vi "RT_MAIN.vi"() -> ()   [LabVIEW 2019]
uses:
  <vilib>/rvi/interface/nirviOpenFPGA/nirviOpenFPGA.xnode
  <vilib>/rvi/interface/nirviMethod/nirviMethod.xnode
  <vilib>/FPGAPlugInAG/Dynamic/niLvFpga_Reset_Dynamic.vi
  <vilib>/FPGAPlugInAG/Dynamic/niLvFpga_Run_Dynamic.vi
  <vilib>/Platform/TimedLoop/XDataNode/XDataNode.xnode
  <vilib>/Platform/TimedLoop/XDataNode/nitl_modes.ctl
  <vilib>/Platform/TimedLoop/XDataNode/XDNodeRunTimeDep.lvlib
  <vilib>/Platform/TimedLoop/XDataNode/wakeup.ctl
  <vilib>/Platform/TimedLoop/XDataNode/timing_clust.ctl
  <vilib>/NI_Real-Time Target Support.lvlib
  <vilib>/FPGAPlugInAG/Dynamic/niLvFpga_Abort_Dynamic.vi
  <vilib>/rvi/interface/nirviCloseFPGA/nirviCloseFPGA.xnode
  ELMO/Elmo Status.ctl
  <vilib>/rvi/interface/nirviReadWriteControl/nirviReadWriteControl.xnode
  <vilib>/Utility/error.llb/Error Cluster From Error Code.vi
  <vilib>/rvi/interface/Simulation/niFpgaSimulationCallBeginRW.vi
  <vilib>/rvi/errors/niLvFpgaAdjustHostInterfaceError.vi
  NiFpgaLv.dll
  <vilib>/Analysis/NI_AALPro.lvlib
  <vilib>/Analysis/5stat.llb/RMS (DBL).vi
  <vilib>/FPGAPlugInAG/Dynamic/niLvFpga_Close_Dynamic.vi
  FPGA Bitfiles/hipabfccurrentpd_FPGATarget_FPGADATA_BIuapcLYHzU.lvbitx
  FPGA/FPGA_DATA.vi
  <vilib>/FPGAPlugInAG/cRIO-9040/niLvFpga_Open_cRIO-9040.vi
  <vilib>/rvi/interface/common/dynamic/niFpgaDynamicAddResources.vi
panel:
  in  "threshold":T1={"High 검출값"=400.0, "Low 기준값"=-400.0, "MID 중간값"=-200.0}
  out "Q_gcp":i32
  out "Control state":string
  in  "문자열":string="system_211111_"
  out "Initial_IMU_R":sgl
  out "Initial_IMU_L":sgl
  out "GCP_R":sgl(slide) scale=0.0..100.0
  out "R_NUM":u32
  in  "Sync Q":bool
  in  "Profile":enum16{"p0", "p1", "p2", "p3", "p4"}(ring)
  in  "Force_peak_control":sgl=300.0
  out "웨이브폼 차트 4":T2(graph)
  out "웨이브폼 차트 3":dbl(graph)
  out "큐의 원소 개수 2":i32
  out "큐의 원소 개수":i32
  out "Q_PSD":i32
  in  "Tuning  2":bool
  out "웨이브폼 차트 2":T3(graph)
  in  "Base force":sgl
  in  "Force_peak":sgl
  in  "ILC coefficient":sgl=0.01
  out "웨이브폼 차트":T3(graph)
  out "Q_motor":i32
  out "Q_data":i32
  out "Q_motor":i32
  out "Status_PS":string
  out "Control param In":T4
  in  "Current Limid 1":cluster{"output high":dbl, "output low":dbl}={"output high"=2885.0, "output low"=-2885.0} {"output high" format="%.2f"; "output low" format="%.2f"}
  in  "Force PD":T5={"proportional gain (Kc)"=15.0, "integral time (Ti, min)"=0.0, "derivative time (Td, min)"=0.0001700000000000005} caption="Force PD 1" {"proportional gain (Kc)" format="%.7f"; "integral time (Ti, min)" format="%.7f"; "derivative time (Td, min)" format="%.7f"}
  in  "2 On/ 1 Off 2":bool
  in  "Motor 0 on / 1 off 2":bool
  in  "PID Set Time(ms) 2":i32
  in  "Force PD":cluster{"(Kp)":dbl, "(Ti)":dbl, "(Td)":dbl}={"(Kp)"=15.0, "(Ti)"=0.0, "(Td)"=0.0002} caption="Force PD 0" {"(Kp)" format="%.7f"; "(Ti)" format="%.7f"; "(Td)" format="%.7f"}
  in  "Current Limd 0":cluster{"output high":dbl, "output low":dbl}={"output high"=2885.0, "output low"=-2885.0} {"output high" format="%.2f"; "output low" format="%.2f"}
  out "A_vel_1":i32
  out "A_pos_1":i32
  out "A Vel_0":i32
  out "A_Pos_0":i32
  out "Motor state":T6(ring)
  in  "SAVE":bool
  out "CPU_LOAD_0 (%)":dbl format="%#_3g"
  out "CPU_LOAD_1 (%)":dbl format="%#_3g"
  in  "STOP":bool
  # "0이 오른쪽 \n1이 왼쪽"
  # "15\n0.0002"
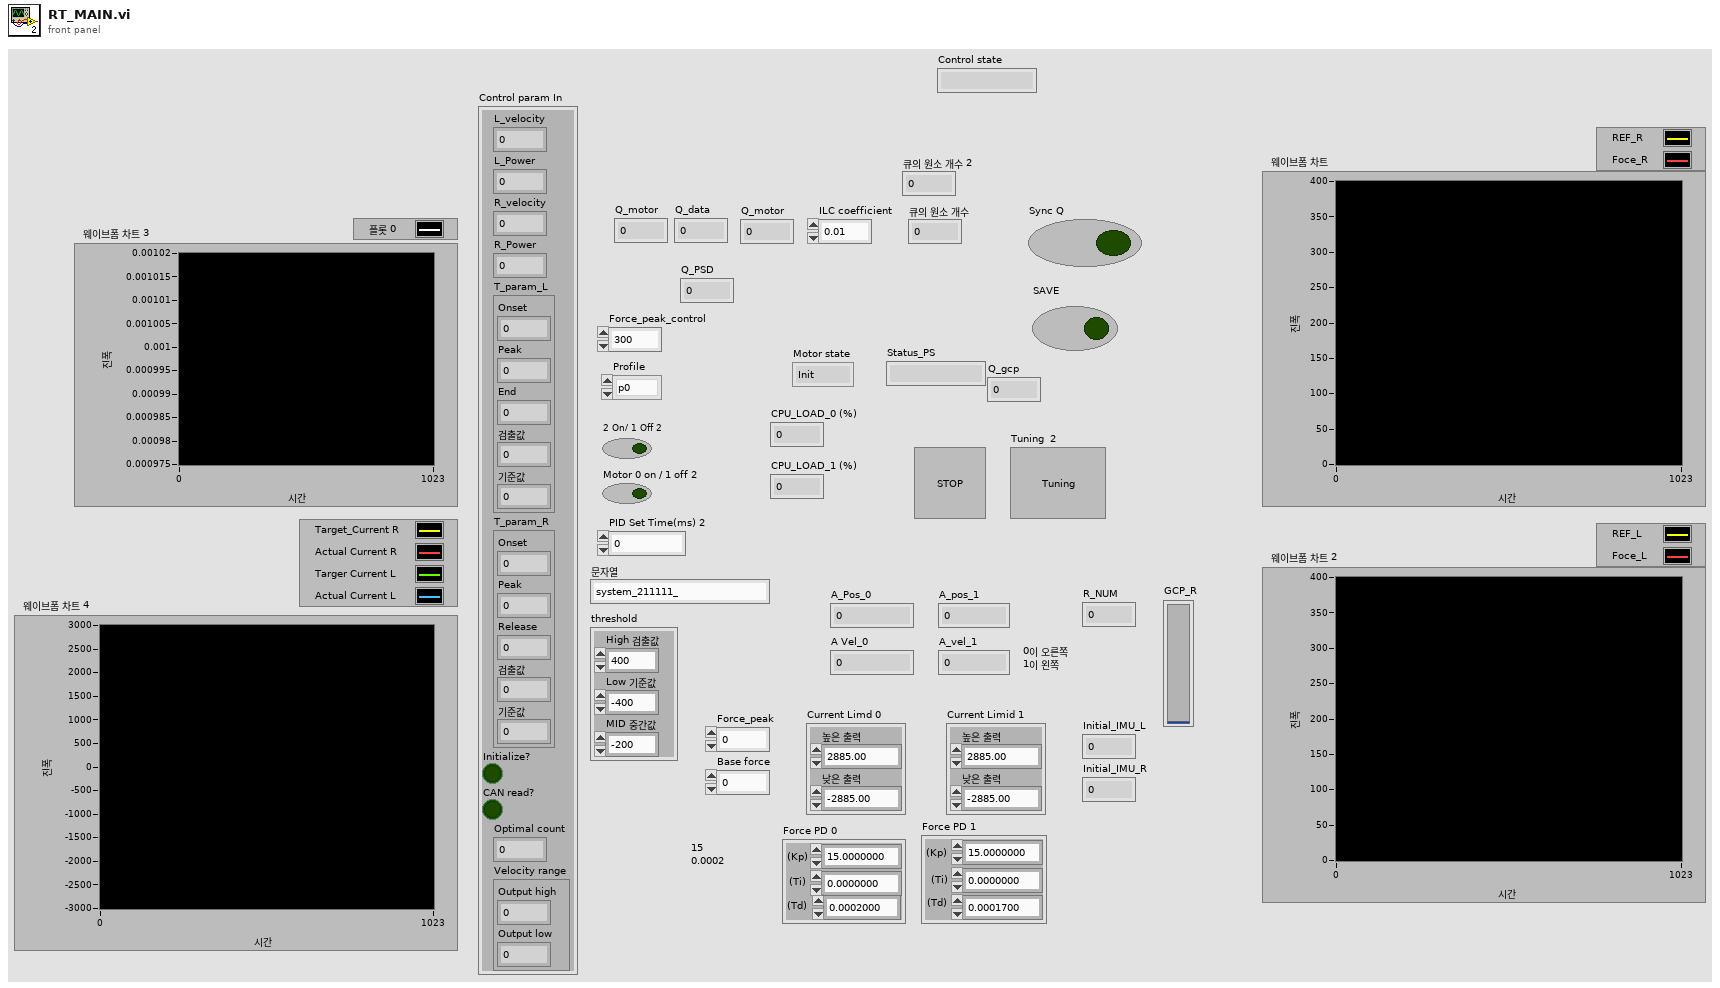
[diagram p1: front panel]
types:
  T1 = cluster{"High 검출값":sgl, "Low 기준값":sgl, "MID 중간값":sgl}
  T2 = cluster{"current_R":i32, "Target Pos_0":i32, "current_L":i32, "Target Pos_0":i32}
  T3 = cluster{"Reference force R":dbl, "Reference force R":dbl}
  T4 = cluster{"L_velocity":u32, "L_Power":sgl, "R_velocity":u32, "R_Power":sgl, "T_param_L":cluster{"Onset":sgl, "Peak":sgl, "End":sgl, "검출값":sgl, "기준값":sgl}, "T_param_R":cluster{"Onset":sgl, "Peak":sgl, "Release":sgl, "검출값":sgl, "기준값":sgl}, "Initialize?":bool, "CAN read?":bool, "Optimal count":i32, "Velocity range":cluster{"Output high":dbl, "Output low":dbl}}
  T5 = cluster{"proportional gain (Kc)":dbl, "integral time (Ti, min)":dbl, "derivative time (Td, min)":dbl}
  T6 = enum16{"Init", "ChkRdy", "Snyc", "Tuning", "Manual"}
  T7 = typedef "XDNodeRunTimeDep.lvlib/timing_clust.ctl" = cluster{"Expected End [f-1]":u64, "Actual End [f-1]":u64, "Finished Late? [f-1]":bool, "Expected End [i-1]":u64, "Actual End [i-1]":u64, "Finished Late? [i-1]":bool, "Expected Start [i]":u64, "Actual Start [i]":u64, "Expected Start [f]":u64, "Actual Start [f]":u64, "Source Name":string, "Structure Name":string, "Period":i64, "Deadline":i64, "Offset":i64, "Start":i64, "Priority":i32, "Timeout":i32, "Mode":T8, "Wakeup Reason":T9, "Error":errorcluster, "Source Type":string, "Secondary Source Type":string, "Global End Time":u64, "Global Start Time":u64, "Frame Duration":u64, "Iteration Duration":u64, "Assigned CPU":i32, "I/O Scan Engine Mode":u32}
  T8 = typedef "XDNodeRunTimeDep.lvlib/nitl_modes.ctl" = enum32{"No Change", "Process missed periods, maintain original phase", "Discard missed periods, maintain original phase", "Process missed periods, ignore original phase", "Discard missed periods, ignore original phase"}
  T9 = typedef "XDNodeRunTimeDep.lvlib/wakeup.ctl" = enum32{"Normal", "Aborted", "Asynchronous wakeup", "Timing source error", "Timed loop error", "Timeout"}
  T10 = typedef "Elmo Status.ctl" = enum16{"Not ready to switch on", "Switch on disabled", "Ready to switch on", "Switch on", "Operation Enabled", "Quick stop active", "Fault reaction active", "Fault", "None"}
  T11 = enum16{"open", "replace", "create", "open or create", "replace or create", "replace or create with confirmation"}
  T12 = cluster{"R_angvel_raw":sgl, "R_angvel_filt":sgl, "L_angvel_raw":sgl, "L_angvel_filt":sgl, "Q_GCP":cluster{"L_num":u32, "L_GCP":dbl, "L_Period":u32, "R_num":u32, "R_GCP":dbl, "R_Period":u32, "L_Ctrl_St":bool, "R_Ctrl_St":bool}}
  T13 = cluster{"L_num":u32, "L_GCP":dbl, "L_Period":u32, "R_num":u32, "R_GCP":dbl, "R_Period":u32, "L_Ctrl_St":bool, "R_Ctrl_St":bool}
  T14 = cluster{"LOAD_CELL_PEAK_L":sgl[], "LOAD_CELL_PEAK_R":sgl[], "Flag_L":enum16{"Release_start", "Calculate", "Onset_start", "Peak_start"}, "Flag_R":enum16{"Release_start", "Calculate", "Onset_start", "Peak_start"}, "Status_PS":string, "GCP_1k_R":sgl, "GCP_1k_L":sgl}
  T15 = cluster{"Actual Pos_0":i32, "Actual Vel_0":i32, "Target Cur_0":i32, "Actual Cur_0":i32, "Actual Pos_1":i32, "Actual Vel_1":i32, "Target Cur_1":i32, "Actual Cur_1":i32, "status_0 ":u16, "status_1":u16}
  T16 = cluster{"Num_L":u32, "Period_L":u32, "GCP_L":sgl, "Num_R":u32, "Period_R":u32, "GCP_R":sgl, "FPGA_Data":sgl[], "L_RUN_OK":bool, "R_RUN_OK":bool, "L_ctrl_start":bool, "R_ctrl_start":bool, "Loop time":dbl, "Integrated time":dbl, "Mode":enum16{"Negative", "Positive", "Full"}}
  T17 = cluster{"Status_PS":string, "Q to xsensor":bool, "FPGA_data":sgl[], "R_force":sgl, "L_force":sgl, "Param":cluster{"Init_Onset_Load":sgl, "Pos_base_L":sgl, "Pos_base_R":sgl, "Init_Vel":i32, "Init_Accel":u32, "Test_Vel":i32, "Test_Acc":u32, "Load_Warning":sgl, "Load_Alarm":sgl, "Control param In":cluster{"L_velocity":u32, "L_Power":sgl, "R_velocity":u32, "R_Power":sgl, "T_param_L":cluster{"Onset":sgl, "Peak":sgl, "End":sgl, "검출값":sgl, "기준값":sgl}, "T_param_R":cluster{"Onset":sgl, "Peak":sgl, "Release":sgl, "검출값":sgl, "기준값":sgl}, "Initialize?":bool, "CAN read?":bool, "Optimal count":i32, "Velocity range":cluster{"Output high":dbl, "Output low":dbl}}, "Init_R":bool, "Init_L":bool, "Force_mode_R":bool, "Force mode_L":bool, "GCP_L":sgl, "GCP_R":sgl, "D_Vel_L":sgl, "D_Vel_R":sgl, "D_Cur_L(/1000)":sgl, "D_Cur_R(/1000)":sgl, "Force_reference_L":sgl, "Force_reference_R":sgl, "Initial_IMU_L":sgl, "Initial_IMU_R":sgl, "L_NUM":u32, "L_Period":i16, "R_NUM":u32, "R_Period":i16, "Initialization count":i32, "R_Ctrl_St":bool, "L_Ctrl_St":bool}}
  T18 = cluster{"Cmd":string, "PSD_state":string, "R_NUM":u32, "L_NUM":u32, "Force_ref_R":sgl, "Force_ref_L":sgl, "Force_L":sgl, "Force_R":sgl, "Force_Mode_R ":bool, "Force_Mode_L":bool, "Current range":cluster{"output high":dbl, "output low":dbl}}
  T19 = cluster{"output high":dbl, "output low":dbl, "proportional gain (Kc)":dbl, "integral time (Ti, min)":dbl, "derivative time (Td, min)":dbl, "output high":dbl, "output low":dbl, "proportional gain (Kc)":dbl, "integral time (Ti, min)":dbl, "derivative time (Td, min)":dbl}
  T20 = cluster{"Q_motor":cluster{"Actual Pos_0":i32, "Actual Vel_0":i32, "Target Cur_0":i32, "Actual Cur_0":i32, "Actual Pos_1":i32, "Actual Vel_1":i32, "Target Cur_1":i32, "Actual Cur_1":i32, "status_0 ":u16, "status_1":u16}, "Q_PSDtoSAVE":i32, "Q_MOTORtoSAVE":i32, "Save_Loop time":dbl, "Save_Integrated time":dbl, "Process":cluster{"Status_PS":string, "Q to xsensor":bool, "FPGA_data":sgl[], "R_force":sgl, "L_force":sgl, "Param":cluster{"Init_Onset_Load":sgl, "Pos_base_L":sgl, "Pos_base_R":sgl, "Init_Vel":i32, "Init_Accel":u32, "Test_Vel":i32, "Test_Acc":u32, "Load_Warning":sgl, "Load_Alarm":sgl, "Control param In":cluster{"L_velocity":u32, "L_Power":sgl, "R_velocity":u32, "R_Power":sgl, "T_param_L":cluster{"Onset":sgl, "Peak":sgl, "End":sgl, "검출값":sgl, "기준값":sgl}, "T_param_R":cluster{"Onset":sgl, "Peak":sgl, "Release":sgl, "검출값":sgl, "기준값":sgl}, "Initialize?":bool, "CAN read?":bool, "Optimal count":i32, "Velocity range":cluster{"Output high":dbl, "Output low":dbl}}, "Init_R":bool, "Init_L":bool, "Force_mode_R":bool, "Force mode_L":bool, "GCP_L":sgl, "GCP_R":sgl, "D_Vel_L":sgl, "D_Vel_R":sgl, "D_Cur_L(/1000)":sgl, "D_Cur_R(/1000)":sgl, "Force_reference_L":sgl, "Force_reference_R":sgl, "Initial_IMU_L":sgl, "Initial_IMU_R":sgl, "L_NUM":u32, "L_Period":i16, "R_NUM":u32, "R_Period":i16, "Initialization count":i32, "R_Ctrl_St":bool, "L_Ctrl_St":bool}}, "GCP":cluster{"R_angvel_raw":sgl, "R_angvel_filt":sgl, "L_angvel_raw":sgl, "L_angvel_filt":sgl, "Q_GCP":cluster{"L_num":u32, "L_GCP":dbl, "L_Period":u32, "R_num":u32, "R_GCP":dbl, "R_Period":u32, "L_Ctrl_St":bool, "R_Ctrl_St":bool}}, "Q_GCPtoSAVE":i32, "Save_loop":i64}
  T21 = cluster{"Q_motor":cluster{"Actual Pos_0":i32, "Actual Vel_0":i32, "Target Cur_0":i32, "Actual Cur_0":i32, "Actual Pos_1":i32, "Actual Vel_1":i32, "Target Cur_1":i32, "Actual Cur_1":i32, "status_0 ":u16, "status_1":u16}, "Q_PSDtoSAVE":i32, "Q_MOTORtoSAVE":i32, "Save_Loop time":dbl, "Save_Integrated time":dbl, "Process":cluster{"Status_PS":string, "Q to xsensor":bool, "FPGA_data":sgl[], "R_force":sgl, "L_force":sgl, "Param":cluster{"Init_Onset_Load":sgl, "Pos_base_L":sgl, "Pos_base_R":sgl, "Init_Vel":i32, "Init_Accel":u32, "Test_Vel":i32, "Test_Acc":u32, "Load_Warning":sgl, "Load_Alarm":sgl, "Control param In":cluster{"L_velocity":u32, "L_Power":sgl, "R_velocity":u32, "R_Power":sgl, "T_param_L":cluster{"Onset":sgl, "Peak":sgl, "End":sgl, "검출값":sgl, "기준값":sgl}, "T_param_R":cluster{"Onset":sgl, "Peak":sgl, "Release":sgl, "검출값":sgl, "기준값":sgl}, "Initialize?":bool, "CAN read?":bool, "Optimal count":i32, "Velocity range":cluster{"Output high":dbl, "Output low":dbl}}, "Init_R":bool, "Init_L":bool, "Force_mode_R":bool, "Force mode_L":bool, "GCP_L":sgl, "GCP_R":sgl, "D_Vel_L":sgl, "D_Vel_R":sgl, "D_Cur_L(/1000)":sgl, "D_Cur_R(/1000)":sgl, "Force_reference_L":sgl, "Force_reference_R":sgl, "Initial_IMU_L":sgl, "Initial_IMU_R":sgl, "L_NUM":u32, "L_Period":i16, "R_NUM":u32, "R_Period":i16, "Initialization count":i32, "R_Ctrl_St":bool, "L_Ctrl_St":bool}}, "GCP":cluster{"R_angvel_raw":sgl, "R_angvel_filt":sgl, "L_angvel_raw":sgl, "L_angvel_filt":sgl, "Q_GCP":cluster{"L_num":u32, "L_GCP":dbl, "L_Period":u32, "R_num":u32, "R_GCP":dbl, "R_Period":u32, "L_Ctrl_St":bool, "R_Ctrl_St":bool}}, "Q_GCPtoSAVE":i32, "Save_loop":i64}[]
  T22 = cluster{"Init_Onset_Load":sgl, "Pos_base_L":sgl, "Pos_base_R":sgl, "Init_Vel":i32, "Init_Accel":u32, "Test_Vel":i32, "Test_Acc":u32, "Load_Warning":sgl, "Load_Alarm":sgl, "Control param In":cluster{"L_velocity":u32, "L_Power":sgl, "R_velocity":u32, "R_Power":sgl, "T_param_L":cluster{"Onset":sgl, "Peak":sgl, "End":sgl, "검출값":sgl, "기준값":sgl}, "T_param_R":cluster{"Onset":sgl, "Peak":sgl, "Release":sgl, "검출값":sgl, "기준값":sgl}, "Initialize?":bool, "CAN read?":bool, "Optimal count":i32, "Velocity range":cluster{"Output high":dbl, "Output low":dbl}}, "Init_R":bool, "Init_L":bool, "Force_mode_R":bool, "Force mode_L":bool, "GCP_L":sgl, "GCP_R":sgl, "D_Vel_L":sgl, "D_Vel_R":sgl, "D_Cur_L(/1000)":sgl, "D_Cur_R(/1000)":sgl, "Force_reference_L":sgl, "Force_reference_R":sgl, "Initial_IMU_L":sgl, "Initial_IMU_R":sgl, "L_NUM":u32, "L_Period":i16, "R_NUM":u32, "R_Period":i16, "Initialization count":i32, "R_Ctrl_St":bool, "L_Ctrl_St":bool}
  T23 = typedef "NI_Real-Time Target Support.lvlib/RT CPU Load.ctl" = cluster{"Total (%)":dbl, "Time Critical (%)":dbl, "Timed Structures (%)":dbl, "High (%)":dbl, "Above Normal (%)":dbl, "Normal (%)":dbl, "Background (%)":dbl, "Idle (%)":dbl, "ISR (%)":dbl}
  T24 = cluster{"CPU loads[0]":T23, "CPU loads[1]":T23, "CPU loads[2]":T23, "CPU loads[3]":T23, "CPU loads[4]":T23, "CPU loads[5]":T23, "CPU loads[6]":T23, "CPU loads[7]":T23, "CPU loads[8]":T23}
  T25 = cluster{"Reference force_L":dbl, "Reference force R":dbl}
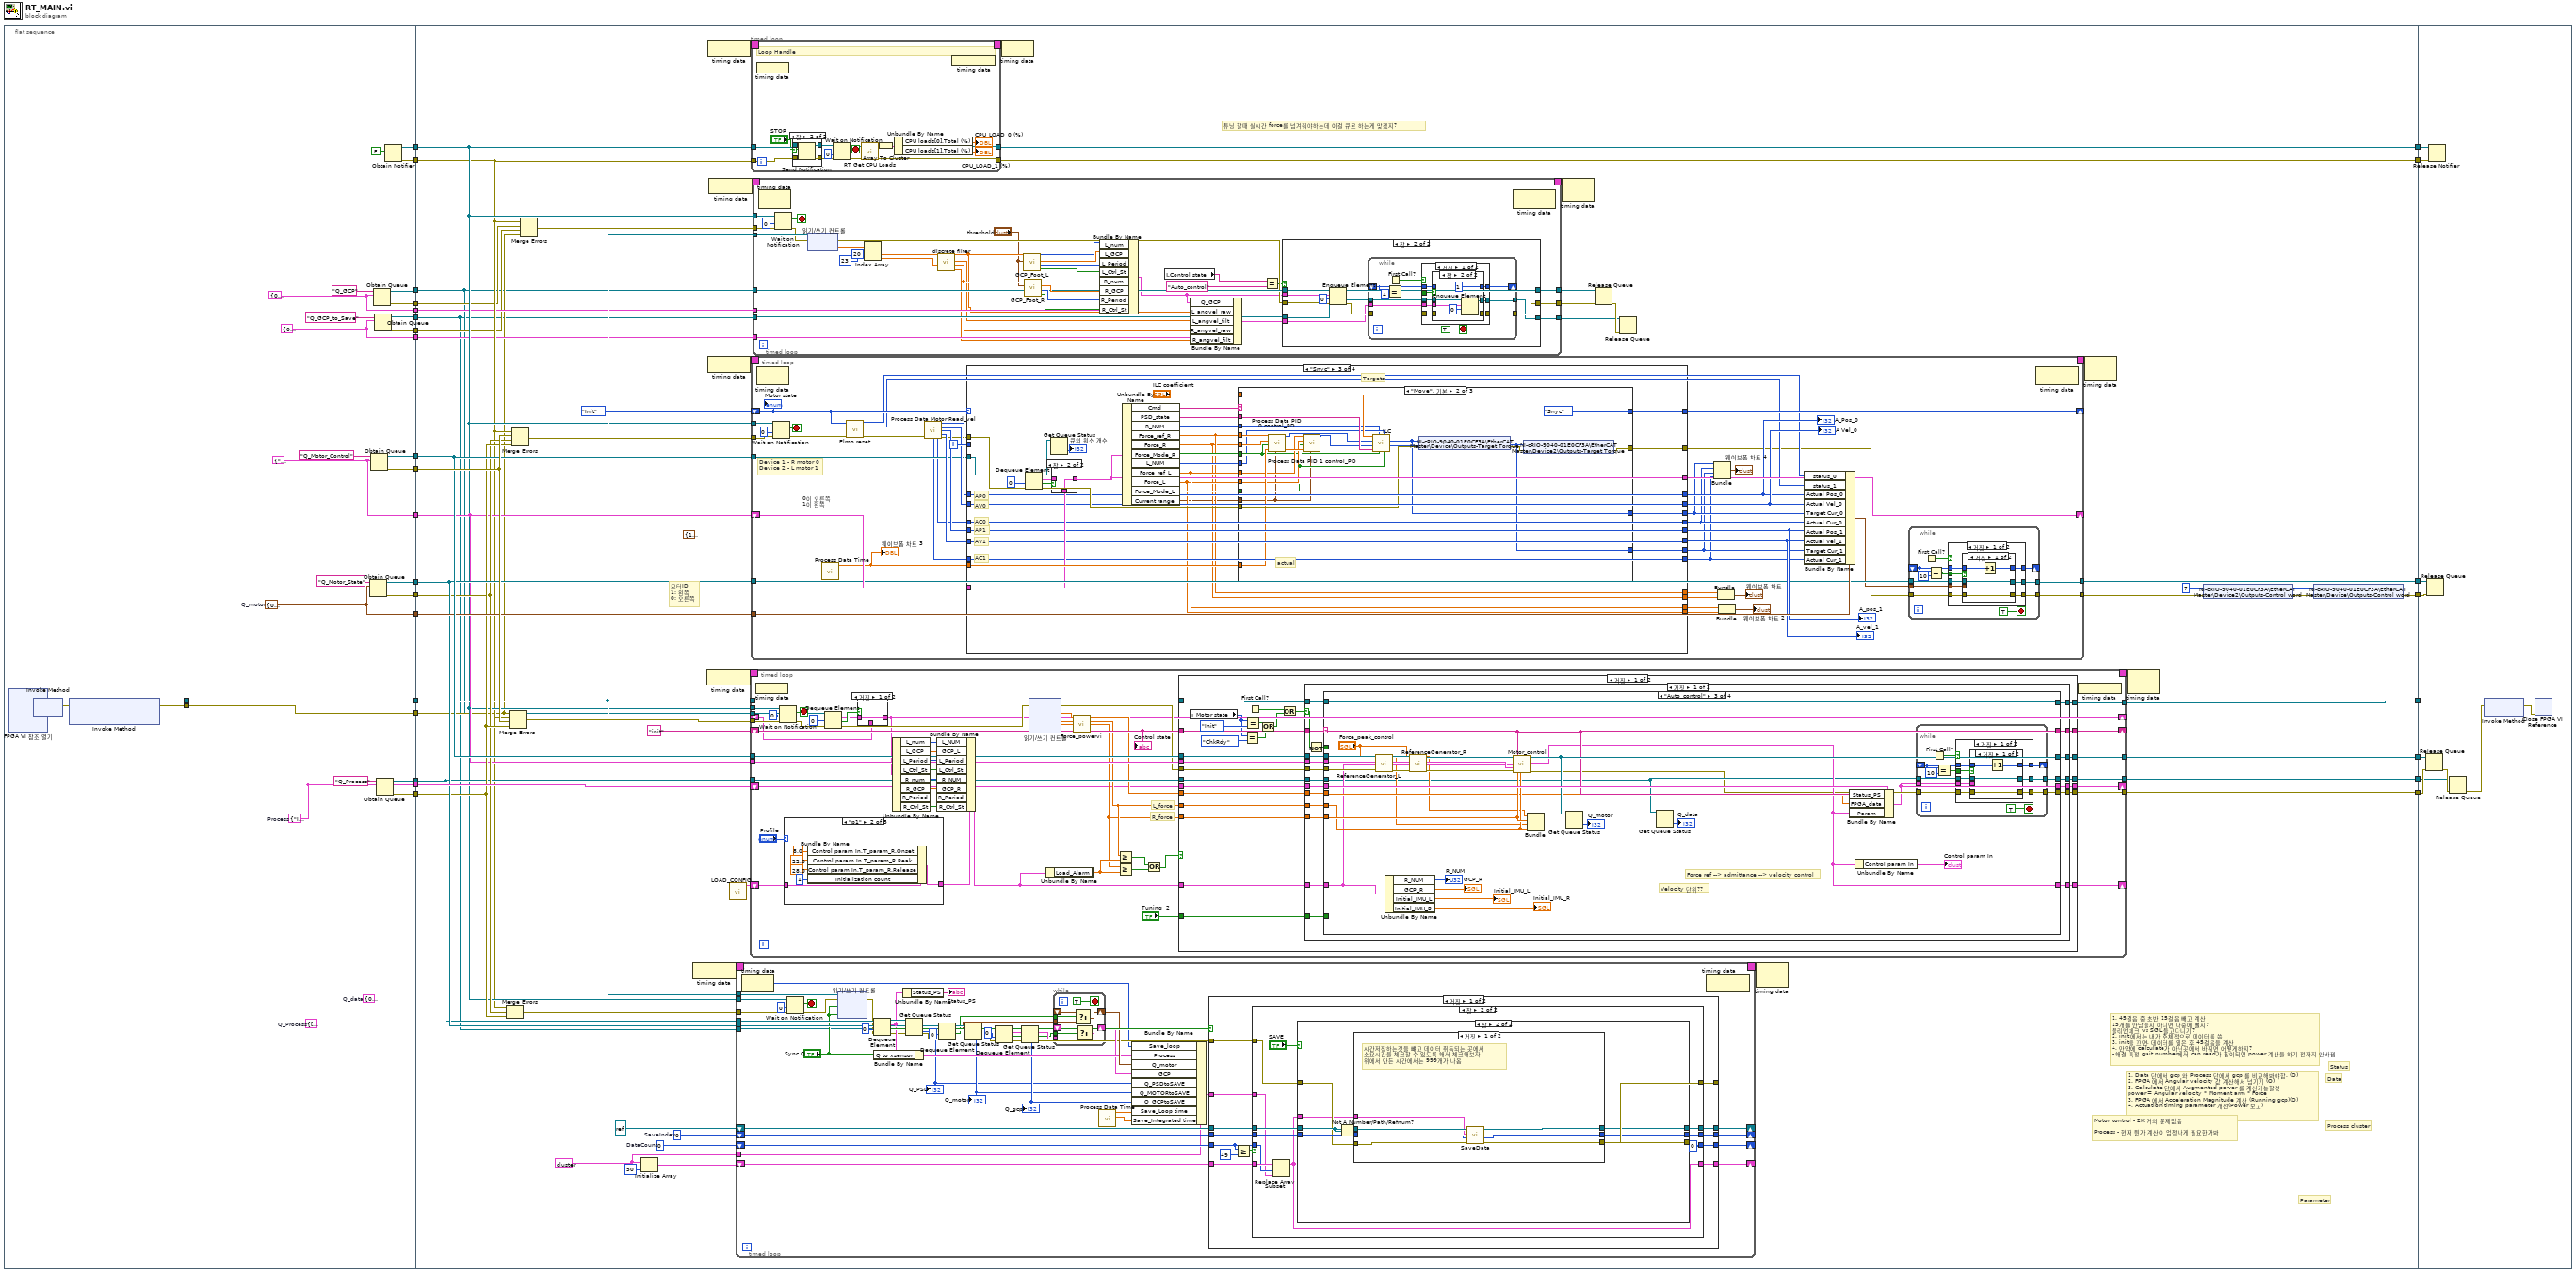
[diagram p0: block diagram]
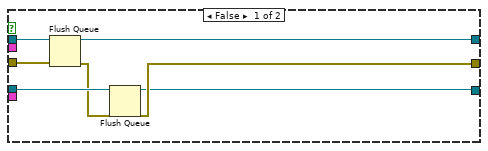
[diagram p2: hidden frame]
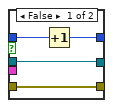
[diagram p3: hidden frame]
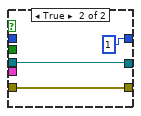
[diagram p4: hidden frame]
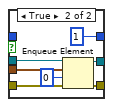
[diagram p6: hidden frame]
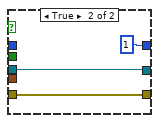
[diagram p7: hidden frame]
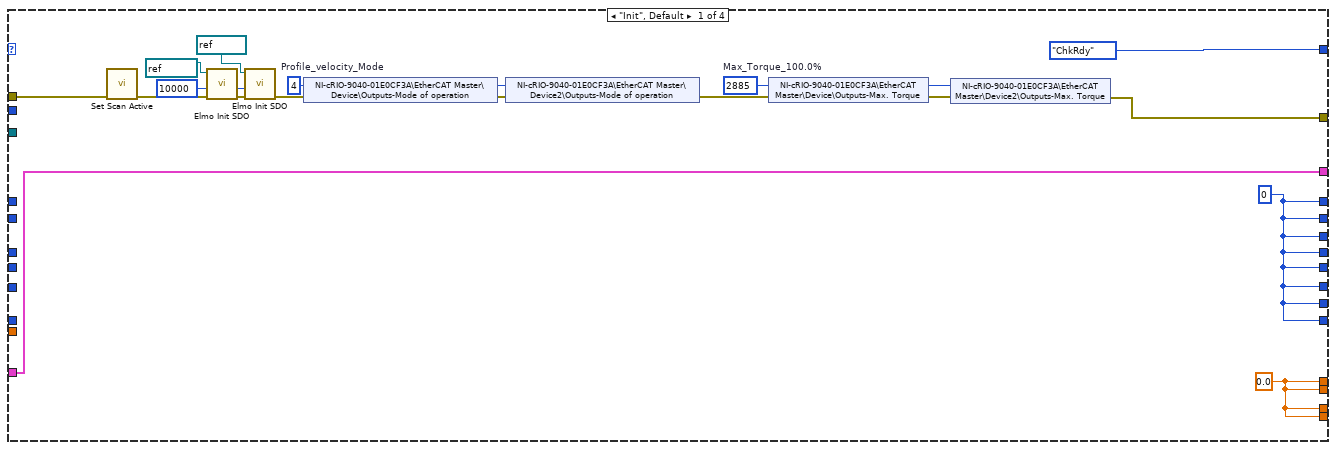
[diagram p8: hidden frame]
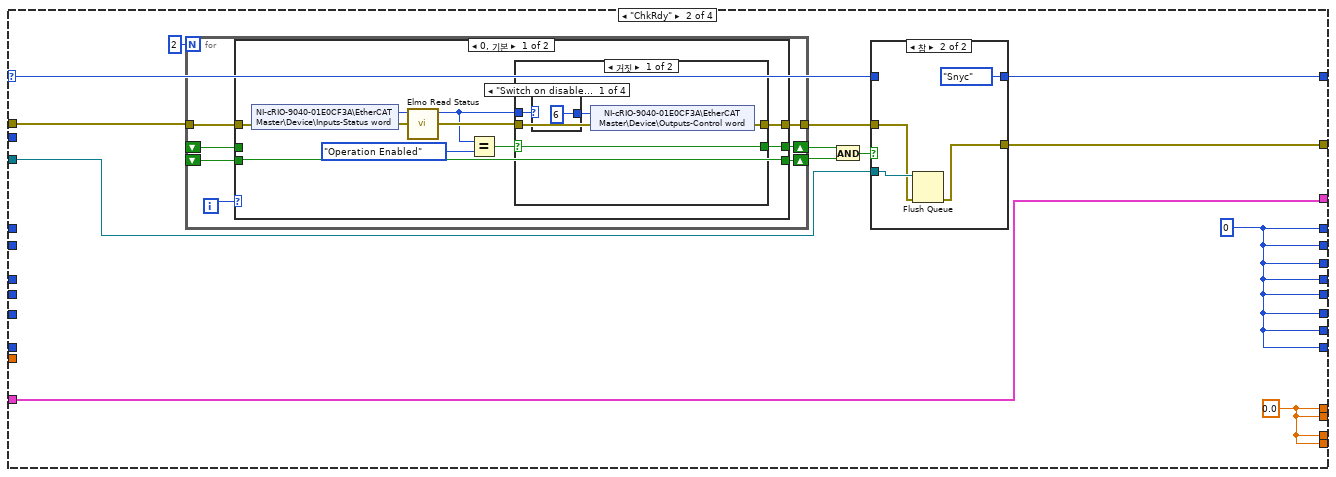
[diagram p9: hidden frame]
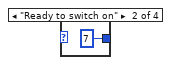
[diagram p10: hidden frame]
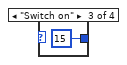
[diagram p11: hidden frame]
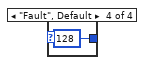
[diagram p12: hidden frame]
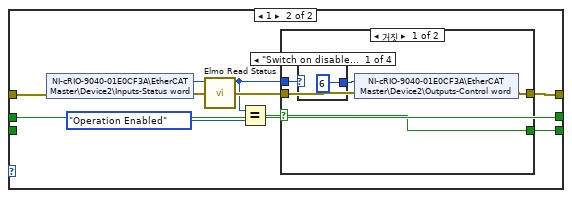
[diagram p14: hidden frame]
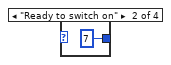
[diagram p15: hidden frame]
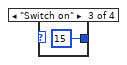
[diagram p16: hidden frame]
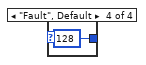
[diagram p17: hidden frame]
diagram:
  n1 = flat-sequence {
    tunnel: [w35] -> w29
    tunnel: [w34] -> w27
    tunnel: w29 -> [w60]
    tunnel: [w60] -> w28
    tunnel: w27 -> [w59]
    tunnel: [w59] -> w26
    tunnel: [w58] -> w25
    tunnel: [w56] -> w24
    tunnel: [w54] -> w20
    tunnel: [w53] -> w19
    tunnel: [w52] -> w18
    tunnel: [w50] -> w16
    tunnel: [w49] -> w15
    tunnel: [w48] -> w14
    tunnel: [w46] -> w10
    tunnel: [w44] -> w9
    tunnel: [w45] -> w7
    tunnel: [w42] -> w6
    tunnel: [w41] -> w5
    tunnel: [w40] -> w4
    tunnel: [w38] -> w3
    tunnel: [w37] -> w2
    tunnel: [w36] -> w1
    tunnel: w28 -> [w75]
    tunnel: w26 -> [w64]
    tunnel: w25 -> [w74]
    tunnel: w24 -> [w73]
    tunnel: [w115] -> w23
    tunnel: [w114] -> w22
    tunnel: [w80] -> w21
    tunnel: w20 -> [w94]
    tunnel: w19 -> [w109]
    tunnel: w18 -> [w79]
    tunnel: [w110] -> w17
    tunnel: w16 -> [w81]
    tunnel: w15 -> [w88]
    tunnel: w14 -> [w107]
    tunnel: [w82] -> w13
    tunnel: [w108] -> w12
    tunnel: [w92] -> w11
    tunnel: w10 -> [w89]
    tunnel: w9 -> [w91]
    tunnel: [w90] -> w8
    tunnel: w7 -> [w87]
    tunnel: w6 -> [w62]
    tunnel: w5 -> [w72]
    tunnel: w4 -> [w71]
    tunnel: w3 -> [w68]
    tunnel: w2 -> [w66]
    tunnel: w1 -> [w61]
    tunnel: w23 -> [w1021]
    tunnel: w22 -> [w1020]
    tunnel: w21 -> [w1019]
    tunnel: w17 -> [w1016]
    tunnel: w13 -> [w1015]
    tunnel: w12 -> [w1011]
    tunnel: w11 -> [w1014]
    tunnel: w8 -> [w1013]
    frame #0 {
      n2 = xnode "FPGA VI 참조 열기"() -> ("FPGA VI 참조 출력"=w31:refnum<k20>, "에러 출력"=w30:errorcluster)  [unwired: 2 in]
      n3 = xnode "Invoke Method"("FPGA VI 참조 입력"=w31, "에러 입력"=w30) -> ("FPGA VI 참조 출력"=w33:refnum<k20>, "에러 출력"=w32:errorcluster)
      n4 = xnode "Invoke Method"("FPGA VI 참조 입력"=w33, "에러 입력"=w32) -> ("FPGA VI 참조 출력"=w35:refnum<k20>, "에러 출력"=w34:errorcluster)  [unwired: 1 in]
    }
    frame #1 {
      w37 = T12 {"R_angvel_raw"=0.0, "R_angvel_filt"=0.0, "L_angvel_raw"=0.0, "L_angvel_filt"=0.0, "Q_GCP"={"L_num"=0, "L_GCP"=0.0, "L_Period"=0, "R_num"=0, "R_GCP"=0.0, "R_Period"=0, "L_Ctrl_St"=FALSE, "R_Ctrl_St"=FALSE}}
      w40 = T13 {"L_num"=0, "L_GCP"=0.0, "L_Period"=0, "R_num"=0, "R_GCP"=0.0, "R_Period"=0, "L_Ctrl_St"=FALSE, "R_Ctrl_St"=FALSE}
      (unwired) T14 {"LOAD_CELL_PEAK_L"=[12.0, 8.0], "LOAD_CELL_PEAK_R"=[], "Flag_L"=enum."Release_start", "Flag_R"=enum."Release_start", "Status_PS"="Init", "GCP_1k_R"=0.0, "GCP_1k_L"=0.0}  # Q_Process
      w44 = T15 {"Actual Pos_0"=0, "Actual Vel_0"=0, "Target Cur_0"=0, "Actual Cur_0"=0, "Actual Pos_1"=0, "Actual Vel_1"=0, "Target Cur_1"=0, "Actual Cur_1"=0, "status_0 "=0, "status_1"=0}  # Q_motor
      (unwired) T16 {"Num_L"=0, "Period_L"=0, "GCP_L"=0.0, "Num_R"=0, "Period_R"=0, "GCP_R"=0.0, "FPGA_Data"=[], "L_RUN_OK"=FALSE, "R_RUN_OK"=FALSE, "L_ctrl_start"=FALSE, "R_ctrl_start"=FALSE, "Loop time"=0.0, "Integrated time"=0.0, "Mode"=enum."Negative"}  # Q_data
      w48 = T17 {"Status_PS"="Init", "Q to xsensor"=FALSE, "FPGA_data"=[0.0, 0.0, 0.0, 0.0, 0.0, 0.0, 0.0, 0.0, 0.0, 0.0, 0.0, 0.0, 0.0, 0.0, 0.0, 0.0, 0.0, 0.0, 0.0, 0.0, 0.0, 0.0, 0.0, 0.0, 0.0, 0.0, 0.0, 0.0, 0.0], "R_force"=0.0, "L_force"=0.0, "Param"={"Init_Onset_Load"=0.0, "Pos_base_L"=0.0, "Pos_base_R"=0.0, "Init_Vel"=0, "Init_Accel"=0, "Test_Vel"=0, "Test_Acc"=0, "Load_Warning"=0.0, "Load_Alarm"=0.0, "Control param In"={"L_velocity"=0, "L_Power"=0.0, "R_velocity"=0, "R_Power"=0.0, "T_param_L"={"Onset"=0.0, "Peak"=0.0, "End"=0.0, "검출값"=0.0, "기준값"=0.0}, "T_param_R"={"Onset"=0.0, "Peak"=0.0, "Release"=0.0, "검출값"=0.0, "기준값"=0.0}, "Initialize?"=FALSE, "CAN read?"=FALSE, "Optimal count"=0, "Velocity range"={"Output high"=0.0, "Output low"=0.0}}, "Init_R"=FALSE, "Init_L"=FALSE, "Force_mode_R"=FALSE, "Force mode_L"=FALSE, "GCP_L"=0.0, "GCP_R"=0.0, "D_Vel_L"=0.0, "D_Vel_R"=0.0, "D_Cur_L(/1000)"=0.0, "D_Cur_R(/1000)"=0.0, "Force_reference_L"=0.0, "Force_reference_R"=0.0, "Initial_IMU_L"=0.0, "Initial_IMU_R"=0.0, "L_NUM"=0, "L_Period"=0, "R_NUM"=0, "R_Period"=0, "Initialization count"=0, "R_Ctrl_St"=FALSE, "L_Ctrl_St"=FALSE}}  # Process
      w52 = T18 {"Cmd"="", "PSD_state"="", "R_NUM"=0, "L_NUM"=0, "Force_ref_R"=0.0, "Force_ref_L"=0.0, "Force_L"=0.0, "Force_R"=0.0, "Force_Mode_R "=FALSE, "Force_Mode_L"=FALSE, "Current range"={"output high"=0.0, "output low"=0.0}}
      n5 = Obtain Queue(name (unnamed)="Q_Motor_State" ("이름(이름없음)"), element data type=w44) -> (queue out=w46:refnum<queue>, error out=w45:errorcluster)  [unwired: 3 in, 1 out]
      n6 = Obtain Queue(name (unnamed)="Q_Motor_Control" ("이름(이름없음)"), element data type=w52) -> (queue out=w54:refnum<queue>, error out=w53:errorcluster)  [unwired: 3 in, 1 out]
      n7 = Obtain Queue(name (unnamed)="Q_GCP" ("이름(이름없음)"), element data type=w40) -> (queue out=w42:refnum<queue>, error out=w41:errorcluster)  [unwired: 3 in, 1 out]
      n8 = Obtain Queue(name (unnamed)="Q_GCP_to_Save" ("이름(이름없음)"), element data type=w37) -> (queue out=w36:refnum<queue>, error out=w38:errorcluster)  [unwired: 3 in, 1 out]
      n9 = Obtain Queue(name (unnamed)="Q_Process" ("이름(이름없음)"), element data type=w48) -> (queue out=w50:refnum<queue>, error out=w49:errorcluster)  [unwired: 3 in, 1 out]
      n10 = Obtain Notifier(notification data type=FALSE ("발견되지 않으면 생성? (참)")) -> (notifier out=w58:refnum<notifier>, error out=w56:errorcluster)  [unwired: 3 in, 1 out]
    }
    frame #2 {
      (unwired) T19 {"output high"=1000000.0, "output low"=-1000000.0, "proportional gain (Kc)"=70.0, "integral time (Ti, min)"=0.0, "derivative time (Td, min)"=0.0, "output high"=1000000.0, "output low"=-1000000.0, "proportional gain (Kc)"=70.0, "integral time (Ti, min)"=0.0, "derivative time (Td, min)"=0.0} ("출력 클러스터")
      w83 = T20 {"Q_motor"={"Actual Pos_0"=0, "Actual Vel_0"=0, "Target Cur_0"=0, "Actual Cur_0"=0, "Actual Pos_1"=0, "Actual Vel_1"=0, "Target Cur_1"=0, "Actual Cur_1"=0, "status_0 "=0, "status_1"=0}, "Q_PSDtoSAVE"=0, "Q_MOTORtoSAVE"=0, "Save_Loop time"=0.0, "Save_Integrated time"=0.0, "Process"={"Status_PS"="Init", "Q to xsensor"=FALSE, "FPGA_data"=[0.0, 0.0, 0.0, 0.0, 0.0, 0.0, 0.0, 0.0, 0.0, 0.0, 0.0, 0.0, 0.0, 0.0, 0.0, 0.0, 0.0, 0.0, 0.0, 0.0, 0.0, 0.0, 0.0, 0.0, 0.0, 0.0, 0.0, 0.0, 0.0], "R_force"=0.0, "L_force"=0.0, "Param"={"Init_Onset_Load"=0.0, "Pos_base_L"=0.0, "Pos_base_R"=0.0, "Init_Vel"=0, "Init_Accel"=0, "Test_Vel"=0, "Test_Acc"=0, "Load_Warning"=0.0, "Load_Alarm"=0.0, "Control param In"={"L_velocity"=0, "L_Power"=0.0, "R_velocity"=0, "R_Power"=0.0, "T_param_L"={"Onset"=0.0, "Peak"=0.0, "End"=0.0, "검출값"=0.0, "기준값"=0.0}, "T_param_R"={"Onset"=0.0, "Peak"=0.0, "Release"=0.0, "검출값"=0.0, "기준값"=0.0}, "Initialize?"=FALSE, "CAN read?"=FALSE, "Optimal count"=0, "Velocity range"={"Output high"=0.0, "Output low"=0.0}}, "Init_R"=FALSE, "Init_L"=FALSE, "Force_mode_R"=FALSE, "Force mode_L"=FALSE, "GCP_L"=0.0, "GCP_R"=0.0, "D_Vel_L"=0.0, "D_Vel_R"=0.0, "D_Cur_L(/1000)"=0.0, "D_Cur_R(/1000)"=0.0, "Force_reference_L"=0.0, "Force_reference_R"=0.0, "Initial_IMU_L"=0.0, "Initial_IMU_R"=0.0, "L_NUM"=0, "L_Period"=0, "R_NUM"=0, "R_Period"=0, "Initialization count"=0, "R_Ctrl_St"=FALSE, "L_Ctrl_St"=FALSE}}, "GCP"={"R_angvel_raw"=0.0, "R_angvel_filt"=0.0, "L_angvel_raw"=0.0, "L_angvel_filt"=0.0, "Q_GCP"={"L_num"=0, "L_GCP"=0.0, "L_Period"=0, "R_num"=0, "R_GCP"=0.0, "R_Period"=0, "L_Ctrl_St"=FALSE, "R_Ctrl_St"=FALSE}}, "Q_GCPtoSAVE"=0, "Save_loop"=0}
      w84 = u16 7 ("Outputs-Control word")
      w103 = 0  # DataCount
      w102 = 0  # SaveIndex
      # "튜닝 할때 실시간 force를 넘겨줘야하는데 이걸 큐로 하는게 맞겠지?"
      # "Motor control - 2K 거의 문제없음\n\nProcess - 현재 뭔가 계산이 엄청나게 필요한가봐"
      # "1. Data 단에서 gcp 와 Process 단에서 gcp 를 비교해봐야함. (O)\n2. FPGA 에서 Angular velocity 값 계산해서 넘기기 (O)\n3. Calculate 단에서 Augmented power 를 계산가능할것\npower = Angular velocity * Moment arm * Force \n3. FPGA 에서 Acceleration Magnitude 계산 (Running gcp)(O)\n4. Actuation timing parameter 개선(Power 보고)"
      # "1. 45걸음 중 초반 15걸음 빼고 계산\n15개를 안담을지 아니면 나중에 뺄지?\n불리언체크 vs SGL 들고다니기? \n2. init 에서는 내가 주체적으로 데이터를 씀 \n3. init을 끄면, 데이터를 읽은 후 45걸음을 계산 \n4. 만약에 calculate가 아닌곳에서 바뀌면 어떻게하지?\n- 해결 특정 gait number에서 can read가 참이되면 power 계산을 하기 전까지 안바뀜"
      # "모터ID \n1: 왼쪽\n0: 오른쪽"
      # "Parameter"
      # "Process cluster"
      # "Status"
      # "Data"
      n11 = Merge Errors(w73, w87, w88) -> (w98:errorcluster)
      n12 = Merge Errors(w64, w73, w109, w88) -> (w111:errorcluster)
      n13 = Merge Errors(w73, w109, w87, w88) -> (w95:errorcluster)
      n14 = Merge Errors(w73, w72, w68, w64) -> (w65:errorcluster)
      n15 = Initialize Array(w83, 50 ("차원 크기")) -> (w99:T21)
      n16 = node-c288() -> (w105:T7)
      n17 = node-c288() -> (w113:T7)
      n18 = node-c288() -> (w117:T7)
      n19 = node-c288() -> (w97:T7)
      n20 = node-c288() -> (w77:T7)
      n21 = call "LOAD_CONFIG.vi"() -> ("출력 클러스터"=w78:T22)  [unwired: 11 in]
      n22 = timed-loop {
        timing: w105 -> [_]
        timing-out: [_] -> w104
        shift-right: [w890] -> _
        shift-left: w102 -> [w893]
        shift-right: [w891] -> _
        shift-left: w103 -> [w894]
        shift-right: [w889] -> _
        shift-left: w99 -> [w892]
        shift-right: [w888] -> _
        shift-left: refnum<file> refnum ("참조 번호 출력") -> [w887]
        tunnel: w74 -> [w885]
        tunnel: w98 -> [w884]
        tunnel: w89 -> [w878]
        tunnel: w81 -> [w883]
        tunnel: w83 -> [w882]
        tunnel: w75 -> [w874]
        tunnel: w61 -> [w868]
        stop <- w895 stop-if-true
        n23 = node-c288() -> (w848:i64)  [unwired: 1 in]
        n24 = Wait on Notification(notifier=w885, timeout in ms (-1)=0 ("타임아웃(ms) (-1)"), error in (no error)=w884) -> (notification=w895:bool, error out=w873:errorcluster)  [unwired: 1 in, 2 out]
        n25 = xnode "읽기/쓰기 컨트롤"("FPGA VI 참조 입력"=w874, "에러 입력"=w873, "DIO1"="Sync Q", "D2"="Sync Q") -> ("에러 출력"=w872:errorcluster)  [unwired: 1 out]
        n26 = Dequeue Element(queue=w883, timeout in ms (-1)=0 ("타임아웃(ms) (-1)"), error in (no error)=w872) -> (queue out=w877:refnum<queue>, element=w876:T17, timed out?=w880:bool, error out=w867:errorcluster)
        n27 = Bundle By Name(cluster=w876, "Q to xsensor"="Sync Q") -> (w856:T17)
        n28 = Unbundle By Name(w876) -> ("Status_PS"=→"Status_PS":string)
        n29 = Get Queue Status(queue=w877, error in (no error)=w867) -> (error out=w866:errorcluster, # elements in queue=w849:i32)  [unwired: 1 in, 6 out]
        "Q_PSD" <- w849
        n30 = Dequeue Element(queue=w878, timeout in ms (-1)=0 ("타임아웃(ms) (-1)"), error in (no error)=w866) -> (queue out=w865:refnum<queue>, element=w861:T15, timed out?=w860:bool, error out=w864:errorcluster)
        n31 = Get Queue Status(queue=w865, error in (no error)=w864) -> (error out=w863:errorcluster, # elements in queue=w850:i32)  [unwired: 1 in, 6 out]
        "Q_motor" <- w850
        n32 = Dequeue Element(queue=w868, timeout in ms (-1)=0 ("타임아웃(ms) (-1)"), error in (no error)=w863) -> (queue out=w852:refnum<queue>, element=w859:T12, timed out?=w858:bool, error out=w853:errorcluster)
        n33 = Get Queue Status(queue=w852, error in (no error)=w853) -> (error out=w854:errorcluster, # elements in queue=w851:i32)  [unwired: 1 in, 6 out]
        "Q_gcp" <- w851
        n34 = while {
          tunnel: w861 -> [w904]
          tunnel: w860 -> [w903]
          shift-right: [w902] -> w857
          shift-left: _ -> [w901]
          tunnel: w859 -> [w899]
          tunnel: w858 -> [w900]
          shift-right: [w898] -> w855
          shift-left: _ -> [w897]
          stop <- TRUE stop-if-true
          n35 = Select(t=w901, s=w903, f=w904) -> (s? t:f=w902:T15)
          n36 = Select(t=w897, s=w900, f=w899) -> (s? t:f=w898:T12)
        }
        n37 = call "Process Data Time.vi"() -> ("Integrated time"=w869:dbl, "Loop time"=w870:dbl)  [unwired: 10 in]
        n38 = Bundle By Name(cluster=w882, "Save_loop"=w848, "Process"=w856, "Q_motor"=w857, "GCP"=w855, "Q_PSDtoSAVE"=w849, "Q_MOTORtoSAVE"=w850, "Q_GCPtoSAVE"=w851, "Save_Loop time"=w870, "Save_Integrated time"=w869) -> (w881:T20)
        n39 = case shown="거짓" w880 {
          tunnel: w854 -> [w915 w999]
          tunnel: w894 -> [w913 w997]
          tunnel: w893 -> [w916 w998]
          tunnel: w892 -> [w914 w996]
          tunnel: [w912 w997] -> w891
          tunnel: [w911 w998] -> w890
          tunnel: [w910 w999] -> _
          tunnel: [w909 w996] -> w889
          tunnel: [w908 w1000] -> w888
          tunnel: w887 -> [w907 w1000]
          tunnel: w881 -> [w906 _]
          frame False {
            n40 = Greater Or Equal?(x=w913, y=49) -> (x >= y?=w917:bool)
            n41 = case shown="참" w917 {
              tunnel: w916 -> [w923 w934]
              tunnel: w915 -> [w922 w932]
              tunnel: w914 -> [w926 w938]
              tunnel: w913 -> [w925 w937]
              tunnel: [w924 0] -> w912
              tunnel: [w923 w933] -> w911
              tunnel: [w922 w929] -> w910
              tunnel: [w921 w928] -> w909
              tunnel: [w920 w931] -> w908
              tunnel: w907 -> [w920 w930]
              tunnel: w906 -> [w919 w927]
              frame False {
                n42 = Replace Array Subset(array=w926, new element=w919, index=w925) -> (w921:T21)
                n43 = Increment(x=w925) -> (x+1=w924:i32)
              }
              frame True {
                n44 = Replace Array Subset(array=w938, new element=w927, index=w937) -> (w928:T21)
                n45 = case shown="참" "SAVE" {
                  tunnel: w934 -> [w944 w955]
                  tunnel: [w944 w950] -> w933
                  tunnel: w932 -> [w943 w954]
                  tunnel: [refnum<file> refnum ("참조 번호") w952] -> w931
                  tunnel: w930 -> [w941 w956]
                  tunnel: w928 -> [_ w953]
                  tunnel: [w939 w951] -> w929
                  frame False {
                    n46 = Not A Number/Path/Refnum?(number/path/refnum=w941) -> (NaN/Path/Refnum?=w940:bool)
                    n47 = case shown="참" w940 {
                      tunnel: [w946 w949] -> w945
                      tunnel: w943 -> [w946 w948]
                      tunnel: w941 -> [_ w947]
                      frame False {
                      }
                      frame True {
                        n48 = Close File(refnum=w947, error in=w948) -> (error out=w949:errorcluster)  [unwired: 1 out]
                      }
                    }
                    n49 = call <vilib>:"Clear Errors.vi"("error in (no error)"=w945) -> ("error out"=w939:errorcluster)  [unwired: 5 in, 1 out]
                  }
                  frame True {
                    n50 = Not A Number/Path/Refnum?(number/path/refnum=w956) -> (NaN/Path/Refnum?=w957:bool)
                    n51 = case shown="거짓" w957 {
                      tunnel: w956 -> [w964 _]
                      tunnel: w955 -> [w959 _]
                      tunnel: w954 -> [w960 w979]
                      tunnel: w953 -> [w958 w965]
                      tunnel: [w963 w970] -> w952
                      tunnel: [w961 w967] -> w951
                      tunnel: [w962 w968] -> w950
                      frame False {
                        # "시간저장하는것을 뺴고 데이터 취득되는 곳에서 \n소요시간을 체크할 수 있도록 해서 체크해보자\n위에서 만든 시간에서는 999개가 나옴"
                        n52 = call "SaveData.vi"("에러 입력"=w960, "Index"=w959, "배열"=w958, "참조번호"=w964) -> ("에러 출력"=w961:errorcluster, "Index 2"=w962:i32, "참조 번호 출력"=w963:refnum<file>)  [unwired: 5 in]
                      }
                      frame True {
                        n53 = Format Date/Time String(time format string (%c)="%Y%m%d_%H%M%S.csv" ("시간 포맷 문자열 (%c)")) -> (date/time string=w984:string)  [unwired: 2 in]
                        n54 = Build Path(base path=path "U:/mmcblk0p1" ("베이스 경로"), name or relative path="ABD_" ("시간 포맷 문자열 (%c)")) -> (appended path=w981:path)
                        n55 = call <vilib>:"Check if File or Folder Exists.vi"("error in (no error)"=w979, "path"=w981) -> ("error out"=w980:errorcluster, "file or folder exists?"=w986:bool, "dup path"=w987:path)  [unwired: 7 in]
                        n56 = case shown="거짓" w986 {
                          tunnel: w987 -> [w993 w995]
                          tunnel: [w992 w995] -> w973
                          tunnel: w980 -> [w991 w994]
                          tunnel: [w990 w994] -> w974
                          frame False {
                            n57 = Create Folder(path (use dialog)=w993, error in=w991) -> (created path=w992:path, error out=w990:errorcluster)  [unwired: 1 in, 1 out]
                          }
                          frame True {
                          }
                        }
                        n58 = Concatenate Strings("문자열", w984) -> (w985:string)
                        n59 = Build Path(base path=w973, name or relative path=w985) -> (appended path=w975:path)
                        n60 = Open/Create/Replace File(file path (use dialog)=w975, error in=w974, operation (0:open)=T11."replace or create" ("동작(0:open)")) -> (refnum out=w972:refnum<file>, error out=w977:errorcluster)  [unwired: 3 in, 1 out]
                        n61 = Write to Text File(file (use dialog)=w972, text="Index,L_Load,R_Load,L_Roll,L_Pitch,L_Yaw,L_accX,L_accY,L_accZ,R_Roll,R_Pitch,R_Yaw,R_accX,R_accY,R_accZ,B_Roll,B_Pitch,B_Yaw,B_accX,B_accY,B_accZ,L_angvel_Rol,L_angvel_Pit,L_angvel_Yaw,R_angvel_Rol,R_angvel_Pit,R_angvel_Yaw,B_angvel_Rol,B_angvel_Pit,B_angvel_Yaw,GCP_L,Num_L,Period_L,GCP_R,Num_R,Period_R,Pos_0,Vel_0,T_cur_0,Pos_1,Vel_1,T_cur_1,R_Onset_ctl,R_Peak_ctl,R_Release_ctl,Q_sync,Optimal_count,Force_ref_L,Force_ref_R,Force_mode_L,Force_mode_R,Actual_Cur_0,Actual_Cur_1,Init_count,R_angvel_raw,R_angvel_filt,L_angvel_raw,L_angvel_filt,L_gcp_G,L_num_G,R_gcp,G,R_num_G,status_0,status_1,Q_PSD,Q_MOTOR,Q_GCP,Time_loop,Time_int,Save_loop" ("텍스트"), error in=w977) -> (refnum out=w971:refnum<file>, error out=w966:errorcluster)  [unwired: 1 in, 1 out]
                        n62 = call "SaveData.vi"("에러 입력"=w966, "Index"=1, "배열"=w965, "참조번호"=w971) -> ("에러 출력"=w967:errorcluster, "Index 2"=w968:i32, "참조 번호 출력"=w970:refnum<file>)  [unwired: 5 in]
                      }
                    }
                  }
                }
              }
            }
          }
          frame True {
          }
        }
        n63 = node-c288() -> ()  [unwired: 1 in, 1 out]
      }
      n64 = timed-loop {
        timing: w113 -> [_]
        timing-out: [_] -> w112
        tunnel: w74 -> [w572]
        tunnel: w111 -> [w570]
        tunnel: w94 -> [w561]
        tunnel: w79 -> [w569]
        tunnel: [w567] -> w110
        shift-right: [w568] -> _
        shift-left: w78 -> [w543]
        tunnel: w81 -> [w566]
        tunnel: [w565] -> w82
        tunnel: [w564] -> w108
        shift-right: [w563] -> _
        shift-left: w107 -> [w542]
        shift-right: [w562] -> _
        shift-left: "init" -> [w560]
        tunnel: w75 -> [w555]
        tunnel: [w552] -> w80
        tunnel: w62 -> [w540]
        shift-right: [w533] -> _
        shift-left: _ -> [w535]
        stop <- w571 stop-if-true
        # "R_force"
        # "L_force"
        n65 = node-c288() -> ()  [unwired: 1 in]
        n66 = Wait on Notification(notifier=w572, timeout in ms (-1)=0 ("타임아웃(ms) (-1)"), error in (no error)=w570) -> (notification=w571:bool, error out=w539:errorcluster)  [unwired: 1 in, 2 out]
        n67 = case shown="\"p1\"" "Profile" {
          tunnel: w543 -> [w576 w582 w585 w591 w597]
          tunnel: [w576 w581 w584 w590 w596] -> w534
          frame "p0", Default {
          }
          frame "p1" {
            n68 = Bundle By Name(cluster=w582, "Control param In.T_param_R.Onset"=sgl 8.0, "Control param In.T_param_R.Peak"=sgl 22.0, "Control param In.T_param_R.Release"=sgl 28.0, "Initialization count"=1) -> (w581:T22)
          }
          frame "p2" {
            n69 = Bundle By Name(cluster=w585, "Control param In.T_param_R.Onset"=sgl 20.0, "Control param In.T_param_R.Peak"=sgl 35.0, "Control param In.T_param_R.Release"=sgl 40.0, "Initialization count"=sgl 2.0 ("Control param In.T_param_R.검출값")) -> (w584:T22)
          }
          frame "p3" {
            n70 = Bundle By Name(cluster=w591, "Control param In.T_param_R.Onset"=sgl 40.0, "Control param In.T_param_R.Peak"=sgl 55.0, "Control param In.T_param_R.Release"=sgl 60.0, "Initialization count"=3) -> (w590:T22)
          }
          frame "p4" {
            n71 = Bundle By Name(cluster=w597, "Control param In.T_param_R.Onset"=sgl 50.0, "Control param In.T_param_R.Peak"=sgl 65.0, "Control param In.T_param_R.Release"=sgl 70.0, "Initialization count"=4) -> (w596:T22)
          }
        }
        n72 = Dequeue Element(queue=w540, timeout in ms (-1)=0 ("타임아웃(ms) (-1)"), error in (no error)=w539) -> (element=w536:T13, timed out?=w537:bool, error out=w538:errorcluster)  [unwired: 1 out]
        n73 = case shown="거짓" w537 {
          tunnel: [w574 w575] -> w533
          tunnel: w536 -> [w574 _]
          tunnel: w535 -> [_ w575]
          frame False {
          }
          frame True {
          }
        }
        n74 = Unbundle By Name(w533) -> ("L_num"=w527:u32, "L_GCP"=w528:dbl, "L_Period"=w529:u32, "L_Ctrl_St"=w524:bool, "R_num"=w530:u32, "R_GCP"=w531:dbl, "R_Period"=w532:u32, "R_Ctrl_St"=w525:bool)
        n75 = Bundle By Name(cluster=w534, "L_NUM"=w527, "GCP_L"=w528, "L_Period"=w529, "L_Ctrl_St"=w524, "R_NUM"=w530, "GCP_R"=w531, "R_Period"=w532, "R_Ctrl_St"=w525) -> (w526:T22)
        n76 = xnode "읽기/쓰기 컨트롤"("FPGA VI 참조 입력"=w555, "에러 입력"=w538) -> ("FPGA VI 참조 출력"=w554:refnum<k20>, "에러 출력"=w553:errorcluster, "IMUS"=w548:sgl[], "L_force"=w550:sgl, "R_force"=w549:sgl)
        n77 = Unbundle By Name(w526) -> ("Load_Alarm"=w557:sgl)
        n78 = call "Force_powervi.vi"("IMUS"=w548, "L_force"=w550, "R_force"=w549) -> ("FPGA_data_out"=w551:sgl[], "L_force_psd"=w547:sgl, "R_force_psd"=w546:sgl)  [unwired: 10 in]
        n79 = Greater Or Equal?(x=w547, y=w557) -> (x >= y?=w558:bool)
        n80 = Greater Or Equal?(x=w546, y=w557) -> (x >= y?=w556:bool)
        n81 = Or(x=w558, y=w556) -> (x .or. y?=w559:bool)
        n82 = case shown="거짓" w559 {
          tunnel: w553 -> [w627 w844]
          tunnel: w526 -> [w614 w834]
          tunnel: w561 -> [w617 w825]
          tunnel: w569 -> [w626 w831]
          tunnel: [w625 w845] -> w565
          tunnel: [w624 w840] -> w567
          tunnel: [w623 w834] -> w568
          tunnel: w566 -> [w622 w843]
          tunnel: w542 -> [w621 w839]
          tunnel: [w620 w842] -> w564
          tunnel: [w612 w839] -> w563
          tunnel: [w619 w829] -> w562
          tunnel: w560 -> [w618 w829]
          tunnel: w547 -> [w616 w833]
          tunnel: w546 -> [w615 w832]
          tunnel: w554 -> [w613 w835]
          tunnel: w551 -> [w611 w836]
          tunnel: [w610 w835] -> w552
          tunnel: "Tuning  2" -> [w609 _]
          frame False {
            n83 = local read "Motor state"() -> (w603:T6)
            n84 = Equal?(x=w603, y=T6."ChkRdy") -> (x = y?=w602:bool)
            n85 = Equal?(x=w603, y=T6."Init") -> (x = y?=w605:bool)
            n86 = First Call?() -> (First Call?: T/F=w607:bool)
            n87 = Or(x=w605, y=w602) -> (x .or. y?=w601:bool)
            n88 = Or(x=w607, y=w601) -> (x .or. y?=w606:bool)
            n89 = case shown="거짓" w606 {
              selector: w606 -> [w632 _]
              tunnel: w627 -> [w648 w820]
              tunnel: w626 -> [w647 _]
              tunnel: [w646 w823] -> w625
              tunnel: [w645 w820] -> w624
              tunnel: [w644 w819] -> w623
              tunnel: w622 -> [w643 w822]
              tunnel: w621 -> [w642 w821]
              tunnel: [w641 w822] -> w620
              tunnel: [w639 "init"] -> w619
              tunnel: w618 -> [w638 _]
              tunnel: w617 -> [w637 w823]
              tunnel: w616 -> [w636 _]
              tunnel: w615 -> [w635 _]
              tunnel: w614 -> [w634 w819]
              tunnel: w613 -> [w633 w818]
              tunnel: [w640 w821] -> w612
              tunnel: w611 -> [w630 _]
              tunnel: [w629 w818] -> w610
              tunnel: w609 -> [w628 _]
              frame False {
                n90 = Not(x=w632) -> (.not. x?=w631:bool)
                n91 = case shown="\"Auto_control\"" w638 {
                  selector: w638 -> [w664 w677 w756 _]
                  tunnel: w648 -> [w669 w700 w746 w815]
                  tunnel: w634 -> [w658 w675 w744 w806]
                  tunnel: w637 -> [w660 w703 w760 w816]
                  tunnel: w647 -> [_ w697 w753 w817]
                  tunnel: [w660 w699 w757 w812] -> w646
                  tunnel: [w666 w707 w732 w807] -> w645
                  tunnel: [w654 w675 w739 w806] -> w644
                  tunnel: w643 -> [w668 w709 w735 w810]
                  tunnel: w642 -> [w665 w706 w761 w805]
                  tunnel: [w667 w708 w734 w809] -> w641
                  tunnel: [w665 w706 w731 w797] -> w640
                  tunnel: [w650 w710 w756 w796] -> w639
                  tunnel: w636 -> [_ w684 w754 w799]
                  tunnel: w635 -> [_ w682 w755 w798]
                  tunnel: w631 -> [w661 _ _ _]
                  tunnel: w633 -> [w655 w698 w747 w801]
                  tunnel: w630 -> [w653 w676 w748 w800]
                  tunnel: [w655 w698 w747 w801] -> w629
                  tunnel: w628 -> [w652 w695 _ w804]
                  frame "init", Default {
                    (unwired) "Auto_control"
                    w656 = FALSE ("Force_mode_R")
                    w657 = FALSE ("Init_R")
                    n92 = case shown="참" w661 {
                      tunnel: w669 -> [w670 w674]
                      tunnel: [w670 w671] -> w659
                      frame False {
                      }
                      frame True {
                        w673 = u16 47 ("Outputs-Control word")
                        n93 = shared-variable "NI-cRIO-9040-01E0CF3A\\EtherCAT Master\\Device\\Outputs-Control word"(w673, error in=w674) -> (error out=w672:errorcluster)
                        n94 = shared-variable "NI-cRIO-9040-01E0CF3A\\EtherCAT Master\\Device2\\Outputs-Control word"(w673, error in=w672) -> (error out=w671:errorcluster)
                      }
                    }
                    n95 = Select(t="Tuning", s=w652, f="Search_Onset") -> (s? t:f=w650:string)
                    n96 = Bundle By Name(cluster=w658, "Init_R"=w657, "Init_L"=w657, "Force_mode_R"=w656, "Force mode_L"=w656) -> (w654:T22)
                    n97 = Bundle By Name(cluster=w665, "Status_PS"=w664, "FPGA_data"=w653, "Param"=w654) -> (w663:T17)
                    n98 = Enqueue Element(queue=w668, element=w663, timeout in ms (-1)=0 ("타임아웃(ms) (-1)"), error in (no error)=w659) -> (queue out=w667:refnum<queue>, error out=w666:errorcluster)  [unwired: 1 out]
                  }
                  frame "Search_Onset" {
                    w689 = 2.0
                    n99 = Unbundle By Name(w675) -> ("Init_Onset_Load"=w683:sgl)
                    n100 = Subtract(x=w683, y=w682) -> (x-y=w681:sgl)
                    n101 = Subtract(x=w683, y=w684) -> (x-y=w680:sgl)
                    n102 = Build Array(w680) -> (w686:sgl[])
                    n103 = Bundle By Name(cluster=w697, "PSD_state"=w677, "Cmd"="Move", "Force_ref_L"=w683, "Force_L"=w684, "Force_ref_R"=w683, "Force_R"=w682, "Current range"=cluster{"output high":dbl, "output low":dbl} {"output high"=1000.0, "output low"=-1000.0}) -> (w696:T18)
                    n104 = Build Array(w681) -> (w679:sgl[])
                    n105 = call-poly <vilib>:"RMS.vi"("X"=w686) -> ("rms value"=w691:dbl)  [unwired: 1 out]
                    n106 = call-poly <vilib>:"RMS.vi"("X"=w679) -> ("rms value"=w690:dbl)  [unwired: 1 out]
                    n107 = Less?(x=w691, y=w689) -> (x < y?=w688:bool)
                    n108 = Less?(x=w690, y=w689) -> (x < y?=w687:bool)
                    n109 = And(x=w688, y=w687) -> (x .and. y?=w685:bool)
                    n110 = Enqueue Element(queue=w703, element=w696, timeout in ms (-1)=0 ("타임아웃(ms) (-1)"), error in (no error)=w700) -> (queue out=w699:refnum<queue>, error out=w693:errorcluster)  [unwired: 1 out]
                    n111 = case shown="참" w685 {
                      tunnel: [FALSE w725] -> w678
                      tunnel: w693 -> [w712 w717]
                      tunnel: [w712 w713] -> w692
                      frame False {
                      }
                      frame True {
                        w722 = 100.0
                        n112 = shared-variable "NI-cRIO-9040-01E0CF3A\\EtherCAT Master\\Device\\Inputs-Velocity actual value"(error in=w717) -> (w716:i32, error out=w714:errorcluster)
                        n113 = shared-variable "NI-cRIO-9040-01E0CF3A\\EtherCAT Master\\Device2\\Inputs-Velocity actual value"(error in=w714) -> (w715:i32, error out=w713:errorcluster)
                        n114 = Build Array(w715) -> (w718:i32[])
                        n115 = Build Array(w716) -> (w719:i32[])
                        n116 = call-poly <vilib>:"RMS.vi"("X"=w719) -> ("rms value"=w724:dbl)  [unwired: 1 out]
                        n117 = call-poly <vilib>:"RMS.vi"("X"=w718) -> ("rms value"=w723:dbl)  [unwired: 1 out]
                        n118 = Less?(x=w724, y=w722) -> (x < y?=w721:bool)
                        n119 = Less?(x=w723, y=w722) -> (x < y?=w720:bool)
                        n120 = And(x=w721, y=w720) -> (x .and. y?=w725:bool)
                      }
                    }
                    n121 = case shown="거짓" w695 {
                      tunnel: [w728 "Tuning"] -> w710
                      tunnel: w677 -> [w726 _]
                      tunnel: w678 -> [w727 _]
                      frame False {
                        n122 = Select(t="Auto_control", s=w727, f=w726) -> (s? t:f=w728:string)
                      }
                      frame True {
                      }
                    }
                    n123 = Bundle By Name(cluster=w706, "Status_PS"=w677, "FPGA_data"=w676, "Param"=w675) -> (w705:T17)
                    n124 = Enqueue Element(queue=w709, element=w705, timeout in ms (-1)=0 ("타임아웃(ms) (-1)"), error in (no error)=w692) -> (queue out=w708:refnum<queue>, error out=w707:errorcluster)  [unwired: 1 out]
                  }
                  frame "Auto_control" {
                    # "Velocity 단위??"
                    # "Force ref --> admittance --> velocity control"
                    n125 = call "ReferenceGenerator_L.vi"("Force_peak"="Force_peak_control", "Param In"=w744, "에러 출력"=w746) -> ("Force_Reference_L"=w736:sgl, "Param out"=w742:T22, "에러 출력 2"=w745:errorcluster)  [unwired: 10 in]
                    n126 = Unbundle By Name(w744) -> ("R_NUM"=→"R_NUM":u32, "GCP_R"=→"GCP_R":sgl, "Initial_IMU_L"=→"Initial_IMU_L":sgl, "Initial_IMU_R"=→"Initial_IMU_R":sgl)
                    n127 = call "ReferenceGenerator_R.vi"("Force_peak"="Force_peak_control", "Param In"=w742, "에러 출력"=w745) -> ("Force_ref_R"=w737:sgl, "Param out"=w740:T22, "에러 출력 2"=w741:errorcluster)  [unwired: 10 in]
                    n128 = call "Motor_control.vi"("Q_in"=w760, "Param In"=w740, "클러스터"=w753, "에러 입력(에러 없음)"=w741, "문자열"=w756, "R_force_psd"=w755, "L_force_psd"=w754) -> ("Q_out"=w757:refnum<queue>, "Param out"=w739:T22, "에러 출력"=w733:errorcluster)  [unwired: 10 in]
                    n129 = Bundle("Force_ref_R"=w737, "R_force_psd"=w755, "Force_Reference_L"=w736, "L_force_psd"=w754) -> ()  [unwired: 1 in, 1 out]
                    n130 = Get Queue Status(queue=w757) -> (# elements in queue=→"Q_motor":i32)  [unwired: 2 in, 7 out]
                    n131 = Get Queue Status(queue=w735) -> (# elements in queue=→"Q_data":i32)  [unwired: 2 in, 7 out]
                    n132 = Bundle By Name(cluster=w761, "Status_PS"=w756, "FPGA_data"=w748, "Param"=w739) -> (w731:T17)
                    n133 = Unbundle By Name(w739) -> ("Control param In"=→"Control param In":T4)
                    n134 = while {
                      tunnel: w731 -> [w768]
                      tunnel: w735 -> [w772]
                      tunnel: [w770] -> w734
                      tunnel: w733 -> [w769]
                      tunnel: [w771] -> w732
                      shift-right: [w766] -> _
                      shift-left: _ -> [w765]
                      stop <- TRUE stop-if-true
                      n135 = First Call?() -> (First Call?: T/F=w762:bool)
                      n136 = Equal?(x=w765, y=10) -> (x = y?=w763:bool)
                      n137 = case shown="거짓" w762 {
                        tunnel: w772 -> [w780 w793]
                        tunnel: [w779 w792] -> w771
                        tunnel: [w778 w793] -> w770
                        tunnel: w769 -> [w777 w792]
                        tunnel: w768 -> [w776 _]
                        tunnel: [w775 1] -> w766
                        tunnel: w765 -> [w774 _]
                        tunnel: w763 -> [w773 _]
                        frame False {
                          n138 = case shown="거짓" w773 {
                            tunnel: w780 -> [w784 w791]
                            tunnel: [w783 w790] -> w779
                            tunnel: [w784 w789] -> w778
                            tunnel: w777 -> [w783 w788]
                            tunnel: w776 -> [_ w786]
                            tunnel: [w781 1] -> w775
                            tunnel: w774 -> [w782 _]
                            frame False {
                              n139 = Increment(x=w782) -> (x+1=w781:i32)
                            }
                            frame True {
                              n140 = Enqueue Element(queue=w791, element=w786, timeout in ms (-1)=0 ("타임아웃(ms) (-1)"), error in (no error)=w788) -> (queue out=w789:refnum<queue>, error out=w790:errorcluster)  [unwired: 1 out]
                            }
                          }
                        }
                        frame True {
                        }
                      }
                    }
                  }
                  frame "Tuning" {
                    n141 = Select(t="Tuning", s=w804, f="init") -> (s? t:f=w796:string)
                    n142 = Bundle By Name(cluster=w817, "Cmd"="Tuning", "Force_L"=w799, "Force_R"=w798) -> (w813:T18)
                    n143 = Enqueue Element(queue=w816, element=w813, timeout in ms (-1)=0 ("타임아웃(ms) (-1)"), error in (no error)=w815) -> (queue out=w812:refnum<queue>, error out=w808:errorcluster)  [unwired: 1 out]
                    n144 = Bundle By Name(cluster=w805, "Status_PS"=w796, "FPGA_data"=w800, "L_force"=w799, "R_force"=w798) -> (w797:T17)
                    n145 = Enqueue Element(queue=w810, element=w797, timeout in ms (-1)=0 ("타임아웃(ms) (-1)"), error in (no error)=w808) -> (queue out=w809:refnum<queue>, error out=w807:errorcluster)  [unwired: 1 out]
                  }
                }
              }
              frame True {
              }
            }
          }
          frame True {
            w827 = FALSE ("Force_mode_R")
            w826 = 0 ("M_ID")
            n146 = Bundle By Name(cluster=w831, "Cmd"="Stop", "PSD_state"=w829, "R_NUM"=w826, "L_NUM"=w826, "Force_ref_R"=w826, "Force_ref_L"=w826, "Force_L"=w826, "Force_R"=w826, "Force_Mode_R"=w827, "Force_Mode_L"=w827) -> (w830:T18)
            n147 = Enqueue Element(queue=w825, element=w830, error in (no error)=w844) -> (queue out=w845:refnum<queue>, error out=w841:errorcluster)  [unwired: 1 in, 1 out]
            n148 = Bundle By Name(cluster=w839, "Status_PS"=w829, "FPGA_data"=w836, "L_force"=w833, "R_force"=w832, "Param"=w834) -> (w838:T17)
            n149 = Enqueue Element(queue=w843, element=w838, timeout in ms (-1)=0 ("타임아웃(ms) (-1)"), error in (no error)=w841) -> (queue out=w842:refnum<queue>, error out=w840:errorcluster)  [unwired: 1 out]
          }
        }
        n150 = node-c288() -> ()  [unwired: 1 out]
        "Control state" <- w560
      }
      n151 = timed-loop {
        timing: w117 -> [_]
        timing-out: [_] -> w116
        tunnel: w74 -> [w222]
        tunnel: w73 -> [w220]
        tunnel: [w210] -> w115
        tunnel: [w209] -> w114
        stop <- w216 stop-if-true
        # "Loop Handle"
        n152 = node-c288() -> ()  [unwired: 1 in]
        n153 = case shown="참" "STOP" {
          selector: "STOP" -> [_ w227]
          tunnel: w222 -> [w224 w229]
          tunnel: w220 -> [w223 w228]
          tunnel: [w224 w226] -> w217
          tunnel: [w223 w225] -> w218
          frame False {
          }
          frame True {
            n154 = Send Notification(notification=w227, notifier=w229, error in (no error)=w228) -> (notifier out=w226:refnum<notifier>, error out=w225:errorcluster)
          }
        }
        n155 = Wait on Notification(notifier=w217, timeout in ms (-1)=0 ("타임아웃(ms) (-1)"), error in (no error)=w218) -> (notifier out=w210:refnum<notifier>, notification=w216:bool, error out=w211:errorcluster)  [unwired: 1 in, 1 out]
        n156 = call <vilib>:"RT Get CPU Loads.vi"("error in (no error)"=w211) -> ("error out"=w209:errorcluster, "CPU loads"=w215:T23[])  [unwired: 9 in]
        n157 = Array To Cluster(array=w215) -> (cluster=w214:T24)
        n158 = Unbundle By Name(w214) -> ("CPU loads[0].Total (%)"=→"CPU_LOAD_0 (%)":dbl, "CPU loads[1].Total (%)"=→"CPU_LOAD_1 (%)":dbl)
        n159 = node-c288() -> ()  [unwired: 1 out]
      }
      n160 = timed-loop {
        timing: w97 -> [_]
        timing-out: [_] -> w96
        tunnel: w74 -> [w273]
        tunnel: w95 -> [w272]
        tunnel: w94 -> [w266]
        shift-right: [w271] -> _
        shift-left: T6."Init" -> [w242]
        tunnel: [w234] -> w86
        tunnel: w89 -> [w238]
        tunnel: w91 -> [w260]
        tunnel: [w235] -> w90
        shift-right: [w265] -> _
        shift-left: w79 -> [w264]
        i -> [w274]
        stop <- w276 stop-if-true
        # "Device 1 - R motor 0\nDevice 2 - L motor 1"
        # "0이 오른쪽 \n1이 왼쪽"
        n161 = node-c288() -> ()  [unwired: 1 in, 1 out]
        n162 = Wait on Notification(notifier=w273, timeout in ms (-1)=0 ("타임아웃(ms) (-1)"), error in (no error)=w272) -> (notification=w276:bool, error out=w243:errorcluster)  [unwired: 1 in, 2 out]
        n163 = call "Process Data Time.vi"() -> ("Loop time"=w249:dbl)  [unwired: 10 in, 1 out]
        "웨이브폼 차트 3" <- w249
        n164 = call "Elmo reset.vi"("에러 입력"=w243, "Motor status"=w242) -> ("에러 출력"=w239:errorcluster, "status 1"=w241:u16, "Status 0"=w240:u16)  [unwired: 7 in]
        n165 = call "Process Data Motor Read_vel.vi"("에러 입력(에러 없음)"=w239) -> ("Actual Pos_0"=w270:i32, "Actual Vel_0"=w269:i32, "Actual Pos_1"=w268:i32, "Actual Vel_1"=w267:i32, "Actual_Cur_1"=w261:i16, "Actual_Cur_0"=w262:i16, "에러 출력"=w263:errorcluster)  [unwired: 8 in]
        n166 = case shown="\"Snyc\"" w242 {
          selector: w242 -> [_ w338 _ _]
          tunnel: [T6."ChkRdy" w339 w422 w493] -> w271
          tunnel: w263 -> [w325 w337 w424 w474]
          tunnel: [w315 w327 w420 w494] -> w236
          tunnel: w270 -> [_ _ w405 w492]
          tunnel: w269 -> [_ _ w404 w491]
          tunnel: w274 -> [_ _ _ w486]
          tunnel: w249 -> [_ _ w419 w478]
          tunnel: w266 -> [_ w329 w418 w470]
          tunnel: w268 -> [_ _ w402 w488]
          tunnel: w267 -> [_ _ w401 w487]
          tunnel: [w311 w331 w415 w468] -> w265
          tunnel: w264 -> [w311 w331 w414 w471]
          tunnel: w262 -> [_ _ w403 w490]
          tunnel: w261 -> [_ _ w400 w489]
          tunnel: [w312 w332 w405 w492] -> w258
          tunnel: [w312 w332 w404 w491] -> w259
          tunnel: [w312 w332 w406 w479] -> w248
          tunnel: [w312 w332 w403 w490] -> w247
          tunnel: [w312 w332 w402 w488] -> w257
          tunnel: [w312 w332 w401 w487] -> w256
          tunnel: [w312 w332 w400 w489] -> w244
          tunnel: [w312 w332 w407 w480] -> w245
          tunnel: [w310 w330 w397 w466] -> w255
          tunnel: [w310 w330 w399 w465] -> w253
          tunnel: [w310 w330 w398 w464] -> w252
          tunnel: [w310 w330 w396 w463] -> w254
          frame "Init", Default {
            w310 = 0.0 ("Reference force R")
            w312 = 0 ("Target Pos_0")
            w317 = u16 2885  # Max_Torque_100.0%
            w319 = i8 4  # Profile_velocity_Mode
            w323 = 10000 ("Timeout(Scans)")
            n167 = call "Set Scan Active.vi"("error in (no error)"=w325) -> ("Error Out"=w326:errorcluster)  [unwired: 10 in]
            n168 = call "Elmo Init SDO.vi"("Error In"=w326, "Timeout(Scans)"=w323, "Elmo Driver IO"=refnum<k21> "ni.var.io://ni-crio-9040-01e0cf3a/EtherCAT Master/Device" ("Slave Constant")) -> ("error out"=w322:errorcluster)  [unwired: 8 in]
            n169 = call "Elmo Init SDO.vi"("Error In"=w322, "Timeout(Scans)"=w323, "Elmo Driver IO"=refnum<k21> "ni.var.io://ni-crio-9040-01e0cf3a/EtherCAT Master/Device2" ("Slave Constant")) -> ("error out"=w321:errorcluster)  [unwired: 8 in]
            n170 = shared-variable "NI-cRIO-9040-01E0CF3A\\EtherCAT Master\\Device\\Outputs-Mode of operation"(w319, error in=w321) -> (error out=w320:errorcluster)
            n171 = shared-variable "NI-cRIO-9040-01E0CF3A\\EtherCAT Master\\Device2\\Outputs-Mode of operation"(w319, error in=w320) -> (error out=w316:errorcluster)
            n172 = shared-variable "NI-cRIO-9040-01E0CF3A\\EtherCAT Master\\Device\\Outputs-Max. Torque"(w317, error in=w316) -> (error out=w318:errorcluster)
            n173 = shared-variable "NI-cRIO-9040-01E0CF3A\\EtherCAT Master\\Device2\\Outputs-Max. Torque"(w317, error in=w318) -> (error out=w315:errorcluster)
          }
          frame "ChkRdy" {
            w330 = 0.0 ("Reference force R")
            w332 = 0 ("Target Pos_0")
            n174 = for {
              N: 2 -> [_]
              tunnel: w337 -> [w345]
              tunnel: [w344] -> w328
              shift-right: [w343] -> w335
              shift-left: _ -> [w342]
              shift-right: [w341] -> w334
              shift-left: _ -> [w340]
              i -> [w346]
              n175 = case shown="0, 기본" w346 {
                tunnel: w345 -> [w355 w374]
                tunnel: [w352 w372] -> w344
                tunnel: [w348 w367] -> w343
                tunnel: w342 -> [_ w367]
                tunnel: [w347 w368] -> w341
                tunnel: w340 -> [w347 _]
                frame 0, Default {
                  n176 = shared-variable "NI-cRIO-9040-01E0CF3A\\EtherCAT Master\\Device\\Inputs-Status word"(error in=w355) -> (w354:u16, error out=w353:errorcluster)
                  n177 = call "Elmo Read Status.vi"("State Word"=w354) -> ("Elmo State"=w350:T10)  [unwired: 7 in, 3 out]
                  n178 = Equal?(x=w350, y=Elmo_Status."Operation Enabled" ("Elmo State")) -> (x = y?=w351:bool)
                  n179 = case shown="거짓" w351 {
                    selector: w351 -> [w358 w365]
                    tunnel: w353 -> [w360 w366]
                    tunnel: [w359 w366] -> w352
                    tunnel: w350 -> [w357 _]
                    tunnel: [w358 w365] -> w348
                    frame False {
                      n180 = case shown="\"Switch on disabled\"" w357 {
                        tunnel: [u16 6 u16 7 u16 15 u16 128] -> w356
                        frame "Switch on disabled" {
                        }
                        frame "Ready to switch on" {
                        }
                        frame "Switch on" {
                        }
                        frame "Fault", Default {
                        }
                      }
                      n181 = shared-variable "NI-cRIO-9040-01E0CF3A\\EtherCAT Master\\Device\\Outputs-Control word"(w356, error in=w360) -> (error out=w359:errorcluster)
                    }
                    frame True {
                    }
                  }
                }
                frame 1 {
                  n182 = shared-variable "NI-cRIO-9040-01E0CF3A\\EtherCAT Master\\Device2\\Inputs-Status word"(error in=w374) -> (w375:u16, error out=w373:errorcluster)
                  n183 = call "Elmo Read Status.vi"("State Word"=w375) -> ("Elmo State"=w371:T10)  [unwired: 7 in, 3 out]
                  n184 = Equal?(x=w371, y=Elmo_Status."Operation Enabled" ("Elmo State")) -> (x = y?=w370:bool)
                  n185 = case shown="거짓" w370 {
                    selector: w370 -> [w380 w385]
                    tunnel: w373 -> [w377 w386]
                    tunnel: [w376 w386] -> w372
                    tunnel: w371 -> [w379 _]
                    tunnel: [w380 w385] -> w368
                    frame False {
                      n186 = case shown="\"Switch on disabled\"" w379 {
                        tunnel: [u16 6 u16 7 u16 15 u16 128] -> w378
                        frame "Switch on disabled" {
                        }
                        frame "Ready to switch on" {
                        }
                        frame "Switch on" {
                        }
                        frame "Fault", Default {
                        }
                      }
                      n187 = shared-variable "NI-cRIO-9040-01E0CF3A\\EtherCAT Master\\Device2\\Outputs-Control word"(w378, error in=w377) -> (error out=w376:errorcluster)
                    }
                    frame True {
                    }
                  }
                }
              }
            }
            n188 = And(x=w335, y=w334) -> (x .and. y?=w333:bool)
            n189 = case shown="참" w333 {
              tunnel: [w388 T6."Snyc"] -> w339
              tunnel: w338 -> [w388 _]
              tunnel: w329 -> [_ w391]
              tunnel: w328 -> [w387 w390]
              tunnel: [w387 w389] -> w327
              frame False {
              }
              frame True {
                n190 = Flush Queue(queue=w391, error in (no error)=w390) -> (error out=w389:errorcluster)  [unwired: 2 out]
              }
            }
          }
          frame "Snyc" {
            # "AP0"
            # "AV0"
            # "AC0"
            # "AC1"
            # "AV1"
            # "AP1"
            # "Targets"
            n191 = Dequeue Element(queue=w418, timeout in ms (-1)=0 ("타임아웃(ms) (-1)"), error in (no error)=w424) -> (queue out=w395:refnum<queue>, element=w416:T18, timed out?=w417:bool, error out=w423:errorcluster)
            n192 = Get Queue Status(queue=w395) -> (# elements in queue=→"큐의 원소 개수":i32)  [unwired: 2 in, 7 out]
            n193 = case shown="참" w417 {
              tunnel: w416 -> [w426 _]
              tunnel: [w426 w427] -> w415
              tunnel: w414 -> [_ w427]
              frame False {
              }
              frame True {
              }
            }
            n194 = Unbundle By Name(w415) -> ("Cmd"=w421:string, "PSD_state"=w408:string, "R_NUM"=w409:u32, "Force_ref_R"=w397:sgl, "Force_R"=w396:sgl, "Force_Mode_R"=w410:bool, "L_NUM"=w411:u32, "Force_ref_L"=w399:sgl, "Force_L"=w398:sgl, "Force_Mode_L"=w412:bool, "Current range"=w393:cluster{"output high":dbl, "output low":dbl})
            n195 = case shown="\"Move\", 기본" w421 {
              tunnel: [w430 w452 w457] -> w420
              tunnel: w423 -> [w432 w454 w457]
              tunnel: [T6."ChkRdy" T6."Snyc" T6."Tuning"] -> w422
              tunnel: w419 -> [_ w450 _]
              tunnel: w398 -> [_ w447 _]
              tunnel: "ILC coefficient" -> [_ w451 _]
              tunnel: w412 -> [_ w442 _]
              tunnel: w399 -> [_ w446 _]
              tunnel: w411 -> [_ w439 _]
              tunnel: w410 -> [_ w441 _]
              tunnel: w396 -> [_ w444 _]
              tunnel: w397 -> [_ w443 _]
              tunnel: w409 -> [_ w438 _]
              tunnel: w408 -> [_ w449 _]
              tunnel: [w428 w437 w455] -> w407
              tunnel: [w428 w436 w455] -> w406
              tunnel: w393 -> [_ w434 _]
              frame "Stop" {
                w428 = 0 ("Target_Pos")
                w429 = u16 2 ("Outputs-Control word")
                n196 = shared-variable "NI-cRIO-9040-01E0CF3A\\EtherCAT Master\\Device\\Outputs-Control word"(w429, error in=w432) -> (error out=w431:errorcluster)
                n197 = shared-variable "NI-cRIO-9040-01E0CF3A\\EtherCAT Master\\Device\\Outputs-Control word"(w429, error in=w431) -> (error out=w430:errorcluster)
              }
              frame "Move", Default {
                # "actual"
                n198 = call "Process Data PID 0 control_PD.vi"("output range 2"=w434, "dt IN (s)"=w450, "Froce_mode"=w441, "R_force"=w444, "R_force_Ref"=w443) -> ("dt OUT (s)"=w448:dbl, "Targer Cur R"=w440:i16)  [unwired: 5 in]
                n199 = call "Process Data PID 1 control_PD.vi"("output range"=w434, "dt IN (s)"=w448, "Froce_mode"=w442, "L_force"=w447, "L_force_Ref"=w446) -> ("Targer Cur L"=w445:i16)  [unwired: 5 in, 1 out]
                n200 = call "ILC.vi"("Force_mode_L"=w442, "L_NUM"=w439, "Force_mode_R"=w441, "R_NUM"=w438, "문자열"=w449, "Target_Cur_L"=w445, "Targer_Cur_R"=w440, "ILC coefficient"=w451) -> ("Target_Cur_L"=w437:i32, "Target_cur_R"=w436:i32)  [unwired: 2 in]
                n201 = shared-variable "NI-cRIO-9040-01E0CF3A\\EtherCAT Master\\Device\\Outputs-Target Torque"(w436, error in=w454) -> (error out=w453:errorcluster)
                n202 = shared-variable "NI-cRIO-9040-01E0CF3A\\EtherCAT Master\\Device2\\Outputs-Target Torque"(w437, error in=w453) -> (error out=w452:errorcluster)
              }
              frame "Tuning" {
                w455 = 0 ("Target_cur_R")
              }
            }
          }
          frame "Tuning" {
            n203 = Dequeue Element(queue=w470, timeout in ms (-1)=0 ("타임아웃(ms) (-1)"), error in (no error)=w474) -> (queue out=w458:refnum<queue>, element=w472:T18, timed out?=w475:bool, error out=w473:errorcluster)
            n204 = case shown="참" w475 {
              tunnel: w472 -> [w497 _]
              tunnel: [w497 w498] -> w468
              tunnel: w471 -> [_ w498]
              frame False {
              }
              frame True {
              }
            }
            n205 = Get Queue Status(queue=w458) -> (# elements in queue=→"큐의 원소 개수 2":i32)  [unwired: 2 in, 7 out]
            n206 = Unbundle By Name(w468) -> ("Cmd"=w462:string, "Force_R"=w463:sgl, "Force_L"=w464:sgl)
            n207 = call "Process Data PID 0 Set_PD.vi"("Force_peak"="Force_peak", "Force"=w463, "Base force"="Base force", "dt IN (s)"=w478, "Num"=w486, "PID Set Time(ms)"="PID Set Time(ms) 2", "output range"="Current Limd 0", "PID gains"="Force PD") -> ("current_R"=w479:i32, "Reference force R"=w466:dbl, "dt OUT (s)"=w477:dbl)  [unwired: 9 in]
            n208 = call "Process Data PID 1 Set_PD.vi"("Force_peak"="Force_peak", "Force"=w464, "Base force"="Base force", "dt IN (s)"=w477, "Num"=w486, "PID Set Time(ms)"="PID Set Time(ms) 2", "output range"="Current Limid 1", "PID gains"="Force PD") -> ("current_L"=w480:i32, "Reference force_L"=w465:dbl)  [unwired: 9 in, 1 out]
            n209 = case shown="참" "2 On/ 1 Off 2" {
              tunnel: w473 -> [w503 w514]
              tunnel: w479 -> [w502 w510]
              tunnel: [w501 w512] -> w495
              tunnel: w480 -> [w499 w511]
              frame False {
                n210 = case shown="거짓" "Motor 0 on / 1 off 2" {
                  tunnel: w502 -> [_ w509]
                  tunnel: w503 -> [w506 w508]
                  tunnel: [w505 w507] -> w501
                  tunnel: w499 -> [w504 _]
                  frame False {
                    n211 = shared-variable "NI-cRIO-9040-01E0CF3A\\EtherCAT Master\\Device2\\Outputs-Target Torque"(w504, error in=w506) -> (error out=w505:errorcluster)
                  }
                  frame True {
                    n212 = shared-variable "NI-cRIO-9040-01E0CF3A\\EtherCAT Master\\Device\\Outputs-Target Torque"(w509, error in=w508) -> (error out=w507:errorcluster)
                  }
                }
              }
              frame True {
                n213 = shared-variable "NI-cRIO-9040-01E0CF3A\\EtherCAT Master\\Device\\Outputs-Target Torque"(w510, error in=w514) -> (error out=w513:errorcluster)
                n214 = shared-variable "NI-cRIO-9040-01E0CF3A\\EtherCAT Master\\Device2\\Outputs-Target Torque"(w511, error in=w513) -> (error out=w512:errorcluster)
              }
            }
            n215 = Equal?(x=w462, y="Tuning") -> (x = y?=w460:bool)
            n216 = case shown="거짓" w460 {
              tunnel: [T6."Snyc" T6."Tuning"] -> w493
              tunnel: w495 -> [w517 w520]
              tunnel: [w515 w520] -> w494
              frame False {
                w518 = u16 7 ("Outputs-Control word")
                n217 = shared-variable "NI-cRIO-9040-01E0CF3A\\EtherCAT Master\\Device2\\Outputs-Control word"(w518, error in=w517) -> (error out=w516:errorcluster)
                n218 = shared-variable "NI-cRIO-9040-01E0CF3A\\EtherCAT Master\\Device\\Outputs-Control word"(w518, error in=w516) -> (error out=w515:errorcluster)
              }
              frame True {
              }
            }
          }
        }
        "A_Pos_0" <- w258
        "A Vel_0" <- w259
        "A_pos_1" <- w257
        "A_vel_1" <- w256
        n219 = Bundle("current_R"=w248, "Target Pos_0"=w247, "current_L"=w245, "Target Pos_0"=w244) -> (→"웨이브폼 차트 4":T2)  [unwired: 1 in]
        n220 = Bundle("Reference force R"=w255, "Reference force R"=w254) -> (→"웨이브폼 차트":T3)  [unwired: 1 in]
        n221 = Bundle("Reference force_L"=w253, "Reference force R"=w252) -> (→"웨이브폼 차트 2":T25)  [unwired: 1 in]
        n222 = Bundle By Name(cluster=w260, "status_0"=w240, "status_1"=w241, "Actual Pos_0"=w258, "Actual Vel_0"=w259, "Target Cur_0"=w248, "Actual Cur_0"=w247, "Actual Pos_1"=w257, "Actual Vel_1"=w256, "Target Cur_1"=w245, "Actual Cur_1"=w244) -> (w237:T15)
        n223 = while {
          tunnel: w237 -> [w283]
          tunnel: w238 -> [w287]
          tunnel: [w285] -> w235
          tunnel: w236 -> [w284]
          tunnel: [w286] -> w234
          shift-right: [w281] -> _
          shift-left: _ -> [w280]
          stop <- TRUE stop-if-true
          n224 = First Call?() -> (First Call?: T/F=w277:bool)
          n225 = Equal?(x=w280, y=10) -> (x = y?=w278:bool)
          n226 = case shown="거짓" w277 {
            tunnel: w287 -> [w295 w308]
            tunnel: [w294 w307] -> w286
            tunnel: [w293 w308] -> w285
            tunnel: w284 -> [w292 w307]
            tunnel: w283 -> [w291 _]
            tunnel: [w290 1] -> w281
            tunnel: w280 -> [w289 _]
            tunnel: w278 -> [w288 _]
            frame False {
              n227 = case shown="거짓" w288 {
                tunnel: w295 -> [w299 w306]
                tunnel: [w298 w305] -> w294
                tunnel: [w299 w304] -> w293
                tunnel: w292 -> [w298 w303]
                tunnel: w291 -> [_ w301]
                tunnel: [w296 1] -> w290
                tunnel: w289 -> [w297 _]
                frame False {
                  n228 = Increment(x=w297) -> (x+1=w296:i32)
                }
                frame True {
                  n229 = Enqueue Element(queue=w306, element=w301, timeout in ms (-1)=0 ("타임아웃(ms) (-1)"), error in (no error)=w303) -> (queue out=w304:refnum<queue>, error out=w305:errorcluster)  [unwired: 1 out]
                }
              }
            }
            frame True {
            }
          }
        }
        n230 = node-c288() -> ()  [unwired: 1 in, 1 out]
        "Motor state" <- w242
      }
      n231 = timed-loop {
        timing: w77 -> [_]
        timing-out: [_] -> w76
        tunnel: w75 -> [w151]
        tunnel: w74 -> [w154]
        tunnel: w71 -> [w146]
        tunnel: w62 -> [w140]
        tunnel: [w139] -> w70
        tunnel: [w138] -> w69
        tunnel: w61 -> [w129]
        tunnel: w66 -> [w128]
        tunnel: w65 -> [w123]
        tunnel: [w122] -> w63
        stop <- w152 stop-if-true
        n232 = node-c288() -> ()  [unwired: 1 in, 1 out]
        n233 = Wait on Notification(notifier=w154, timeout in ms (-1)=0 ("타임아웃(ms) (-1)"), error in (no error)=w123) -> (notification=w152:bool, error out=w150:errorcluster)  [unwired: 1 in, 2 out]
        n234 = xnode "읽기/쓰기 컨트롤"("FPGA VI 참조 입력"=w151, "에러 입력"=w150) -> ("에러 출력"=w137:errorcluster, "IMUS"=w149:sgl[])  [unwired: 1 out]
        n235 = Index Array(array=w149, index #1=20 ("인덱스"), index #2=23 ("인덱스")) -> (element #1=w131:sgl, element #2=w130:sgl)
        n236 = call "discrete filter.vi"("R_angvel_raw"=w130, "L_angvel_raw"=w131) -> ("R_angvel_filt"=w126:sgl, "R_angvel_raw"=w127:sgl, "L_angvel_filt"=w125:sgl, "L_angvel_raw"=w121:sgl)  [unwired: 6 in]
        n237 = call "GCP_Foot_L.vi"("threshold"="threshold", "Foot Angular velocity"=w121) -> ("L_Ctrl_Start"=w133:bool, "L_Period"=w143:u32, "L_GCP"=w144:dbl, "L_num"=w145:u32)  [unwired: 6 in]
        n238 = call "GCP_Foot_R.vi"("threshold"="threshold", "Foot Angular velocity"=w127) -> ("R_Ctrl_Start"=w132:bool, "R_Period"=w141:u32, "R_GCP"=w142:dbl, "R_num"=w118:u32)  [unwired: 6 in]
        n239 = Bundle By Name(cluster=w146, "L_num"=w145, "L_GCP"=w144, "L_Period"=w143, "L_Ctrl_St"=w133, "R_num"=w118, "R_GCP"=w142, "R_Period"=w141, "R_Ctrl_St"=w132) -> (w120:T13)
        n240 = local read "Control state"() -> (w134:string)
        n241 = Bundle By Name(cluster=w128, "Q_GCP"=w120, "L_angvel_raw"=w121, "L_angvel_filt"=w125, "R_angvel_raw"=w127, "R_angvel_filt"=w126) -> (w124:T12)
        n242 = Equal?(x=w134, y="Auto_control") -> (x = y?=w136:bool)
        n243 = case shown="참" w136 {
          tunnel: w140 -> [w161 w170]
          tunnel: w120 -> [_ w169]
          tunnel: [w160 w168] -> w139
          tunnel: [w156 w166] -> w138
          tunnel: w137 -> [w159 w167]
          tunnel: w129 -> [w158 w164]
          tunnel: w124 -> [_ w162]
          tunnel: [w155 w165] -> w122
          frame False {
            n244 = Flush Queue(queue=w161, error in (no error)=w159) -> (queue out=w160:refnum<queue>, error out=w157:errorcluster)  [unwired: 1 out]
            n245 = Flush Queue(queue=w158, error in (no error)=w157) -> (queue out=w155:refnum<queue>, error out=w156:errorcluster)  [unwired: 1 out]
          }
          frame True {
            n246 = Enqueue Element(queue=w170, element=w169, timeout in ms (-1)=0 ("타임아웃(ms) (-1)"), error in (no error)=w167) -> (queue out=w168:refnum<queue>, error out=w163:errorcluster)  [unwired: 1 out]
            n247 = while {
              tunnel: w162 -> [w178]
              tunnel: w164 -> [w182]
              tunnel: [w180] -> w165
              tunnel: w163 -> [w179]
              tunnel: [w181] -> w166
              shift-right: [w176] -> _
              shift-left: _ -> [w175]
              stop <- TRUE stop-if-true
              n248 = Equal?(x=w175, y=4) -> (x = y?=w173:bool)
              n249 = First Call?() -> (First Call?: T/F=w172:bool)
              n250 = case shown="거짓" w172 {
                tunnel: w182 -> [w190 w203]
                tunnel: [w189 w202] -> w181
                tunnel: [w188 w203] -> w180
                tunnel: w179 -> [w187 w202]
                tunnel: w178 -> [w186 _]
                tunnel: [w185 1] -> w176
                tunnel: w175 -> [w184 _]
                tunnel: w173 -> [w183 _]
                frame False {
                  n251 = case shown="참" w183 {
                    tunnel: w190 -> [w194 w201]
                    tunnel: [w193 w200] -> w189
                    tunnel: [w194 w199] -> w188
                    tunnel: w187 -> [w193 w198]
                    tunnel: w186 -> [_ w196]
                    tunnel: [w191 1] -> w185
                    tunnel: w184 -> [w192 _]
                    frame False {
                      n252 = Increment(x=w192) -> (x+1=w191:i32)
                    }
                    frame True {
                      n253 = Enqueue Element(queue=w201, element=w196, timeout in ms (-1)=0 ("타임아웃(ms) (-1)"), error in (no error)=w198) -> (queue out=w199:refnum<queue>, error out=w200:errorcluster)  [unwired: 1 out]
                    }
                  }
                }
                frame True {
                }
              }
            }
          }
        }
        n254 = node-c288() -> ()  [unwired: 1 in, 1 out]
      }
      n255 = node-c288(w116) -> ()
      n256 = node-c288(w76) -> ()  [unwired: 1 out]
      n257 = Release Queue(queue=w70, error in (no error)=w69) -> (error out=w67:errorcluster)  [unwired: 1 in, 2 out]
      n258 = Release Queue(queue=w63, error in (no error)=w67) -> ()  [unwired: 1 in, 3 out]
      n259 = node-c288(w104) -> ()  [unwired: 1 out]
      n260 = node-c288(w96) -> ()  [unwired: 1 out]
      n261 = node-c288(w112) -> ()  [unwired: 1 out]
      n262 = shared-variable "NI-cRIO-9040-01E0CF3A\\EtherCAT Master\\Device2\\Outputs-Control word"(w84, error in=w86) -> (error out=w85:errorcluster)
      n263 = shared-variable "NI-cRIO-9040-01E0CF3A\\EtherCAT Master\\Device\\Outputs-Control word"(w84, error in=w85) -> (error out=w92:errorcluster)
    }
    frame #3 {
      n264 = Release Queue(queue=w1015, error in (no error)=w1016) -> (error out=w1012:errorcluster)  [unwired: 1 in, 2 out]
      n265 = Release Queue(queue=w1013, error in (no error)=w1014) -> ()  [unwired: 1 in, 3 out]
      n266 = Release Notifier(notifier=w1021, error in (no error)=w1020) -> ()  [unwired: 1 in, 3 out]
      n267 = Release Queue(queue=w1011, error in (no error)=w1012) -> (error out=w1010:errorcluster)  [unwired: 1 in, 2 out]
      n268 = xnode "Invoke Method"("FPGA VI 참조 입력"=w1019, "에러 입력"=w1010) -> ("FPGA VI 참조 출력"=w1018:refnum<k20>, "에러 출력"=w1017:errorcluster)
      n269 = xnode "Close FPGA VI Reference"("FPGA VI 참조 입력"=w1018, "에러 입력"=w1017) -> ()  [unwired: 1 out]
    }
  }
